vi "AlliGator FLI Dataset Actions.vi"(0 "AlliGator Q Elements":T4[](array[typedef]), 1 "VI in":refnum<vi>, 2 "Script in":bool, 5 "AlliGator IV DVR in":refnum<data-value>, 7 "AlliGator Q Event in":T5=enum."GUI:Idle", 9 "Data":variant, 11 "error in (no error)":errorcluster, 12 "AlliGator Ctrl Refnums":T6) -> (3 "Script out":bool, 4 "Alligator Queue Elements":T4[](array[typedef]), 6 "AlliGator IV DVR out":refnum<data-value>, 10 "[Notebook Message]":T1[](array[typedef]) {"Message Style"."Text Alignment" items=["Left", "Right", "Center"]}, 15 "error out":errorcluster)   [LabVIEW 2021, in "AlliGator Action Engine.lvlib"]
doc: "Processes AlliGator FLI Dataset-related actions."
uses:
  AlliGator Action Engine.lvlib
  AlliGator Internal Variables v2.ctl
  <vilib>/vision/Image Controls.llb/IMAQ Image.ctl
  AlliGator Gate Image Set.ctl
  AlliGator FLI Dataset Type.ctl
  AlliGator Data Series Type.ctl
  AlliGator Dataset Channel.ctl
  AlliGator Gate Arithmetic.ctl
  AlliGator Displayed Image.ctl
  Image/Named ROI Description.ctl
  AlliGator Decay Metadata v3.ctl
  AlliGator Decay Background Subtraction Info.ctl
  AlliGator Baseline Subtraction Method.ctl
  Graphs/XY Graph/XY Graph Plot Shift Parameters.ctl
  Graphs/XY Graph/XY Graph Plot Shift Method.ctl
  AlliGator Decay Extrapolation Parameters.ctl
  Phasor/Calibration Phasor (m, phi).ctl
  Phasor/Phasor Reference Series.ctl
  Phasor/Phasor Calibration Map v2.ctl
  Phasor/Phasor (g, s).ctl
  AlliGator Raw Phasor Plot Data v4.ctl
  Phasor/Phasor Standard Deviation Options.ctl
  AlliGator Phasor Multi-Harmonic Data.ctl
  Phasor/Phasor Harmonic Data.ctl
  AlliGator Decay Fit Options & Parameters v2.ctl
  Fits/IRF(X)PSED/Decay Fit Options v2.ctl
  Fits/Decay Convolution/Decay Model.ctl
  Fits/Residual Type.ctl
  Fits/IRF(X)PSED/Fit Weights Type.ctl
  Fits/Non-linear Fitting Method v2.ctl
  Fits/Fit Calculation Method.ctl
  Fits/Non-linear Fitting Algorithm.ctl
  AlliGator Decay Fit Parameter Constraints 2.ctl
  Fits/IRF(X)PSED/Decay Fit Parameters In List.ctl
  Fits/IRF(X)PSED/MLE Baseline Offset Type.ctl
  AlliGator Decay Preprocessing Parameters.ctl
  Fits/IRF(X)PSED/Decay Fit Parameters & Derived Quantities List.ctl
  AlliGator Parameter Maps Data.ctl
  AlliGator Q Event.ctl
  AlliGator Ctrl Refnums.ctl
  AlliGator Other Ctrl Refnums.ctl
  AlliGator State Indicator.ctl
  AlliGator Main Window Tabs.ctl
  AlliGator Phasor Plot Ctrl Refnums.ctl
  AlliGator Phasor Graph Ctrl Refnums.ctl
  Phasor/Phasor Calibration Type.ctl
  AlliGator Dataset Ctrl Refnums.ctl
  AlliGator Registered Events Ctrl Refnums.ctl
  AlliGator Image Histogram Control Refnums.ctl
  Histograms/Linear Histogram Options.ctl
  Histograms/Histogram Bin Option.ctl
  Histograms/Histogram Bin Position.ctl
  AlliGator Decay Fit Map Control Refnums.ctl
  AlliGator Q Element.ctl
  Notebook/Notebook Message Object.ctl
  Rich Text Box/Text Formatting.ctl
  Rich Text Box/Text Colors.ctl
  AlliGator State Indicators List.ctl
  Alligator Elements Order in Action Stack.ctl
  Graphs/Plot Point Style.ctl
  Graphs/LabVIEW Plot Interpolation.ctl
  AlliGator Channel Arithmetic Action Parameters.ctl
  AlliGator Multi-ROIs Dialog Type.ctl
  Image/Image Control ROI Description.ctl
  5f8aefbb-6789-42e2-90c6-aefb61e4d968.vi
  AlliGator Add Action Array to Stack.vi
  Variant/Variant to Data/Variant to Boolean.vi
  Graphs/XY Graph/XY Graph Add Single Plot with Name.vi
  Variant/Variant to Data/Variant to String.vi
  Image/Image.lvlib
  AlliGator ROIs.lvlib
  Variant/Variant.lvlib
  Variant/Variant to Data/Variant to Data.lvlib
  GUI/GUI.lvlib
  AlliGator Settings.lvlib
  AlliGator Dual-Channel Datasets.lvlib
  AlliGator Python Plugins.lvlib
  Sound/Sound.lvlib
  AlliGator Source Image.lvlib
  AlliGator Scripts.lvlib
  AlliGator IRF.lvlib
  AlliGator GUI.lvlib
  AlliGator Decay Fit.lvlib
  AlliGator Decay Statistics.lvlib
  AlliGator Internal Variables.lvlib
  AlliGator Decay Processing.lvlib
  Error/Error.lvlib
  AlliGator Decay Fit Parameter Map.lvlib
  AlliGator Phasor Graph.lvlib
  Graphs/Graphs.lvlib
  Graphs/XY Graph/XY Graph Add-Ons.lvlib
  Rich Text Box/Rich Text Box.lvlib
  Phasor/Phasor.lvlib
  AlliGator Decay Preprocessing.lvlib
  AlliGator Files.lvlib
  AlliGator Phasor Plot.lvlib
  Fits/Fits.lvlib
  Histograms/Histogram Window.lvlib
  Notebook/Notebook.lvlib
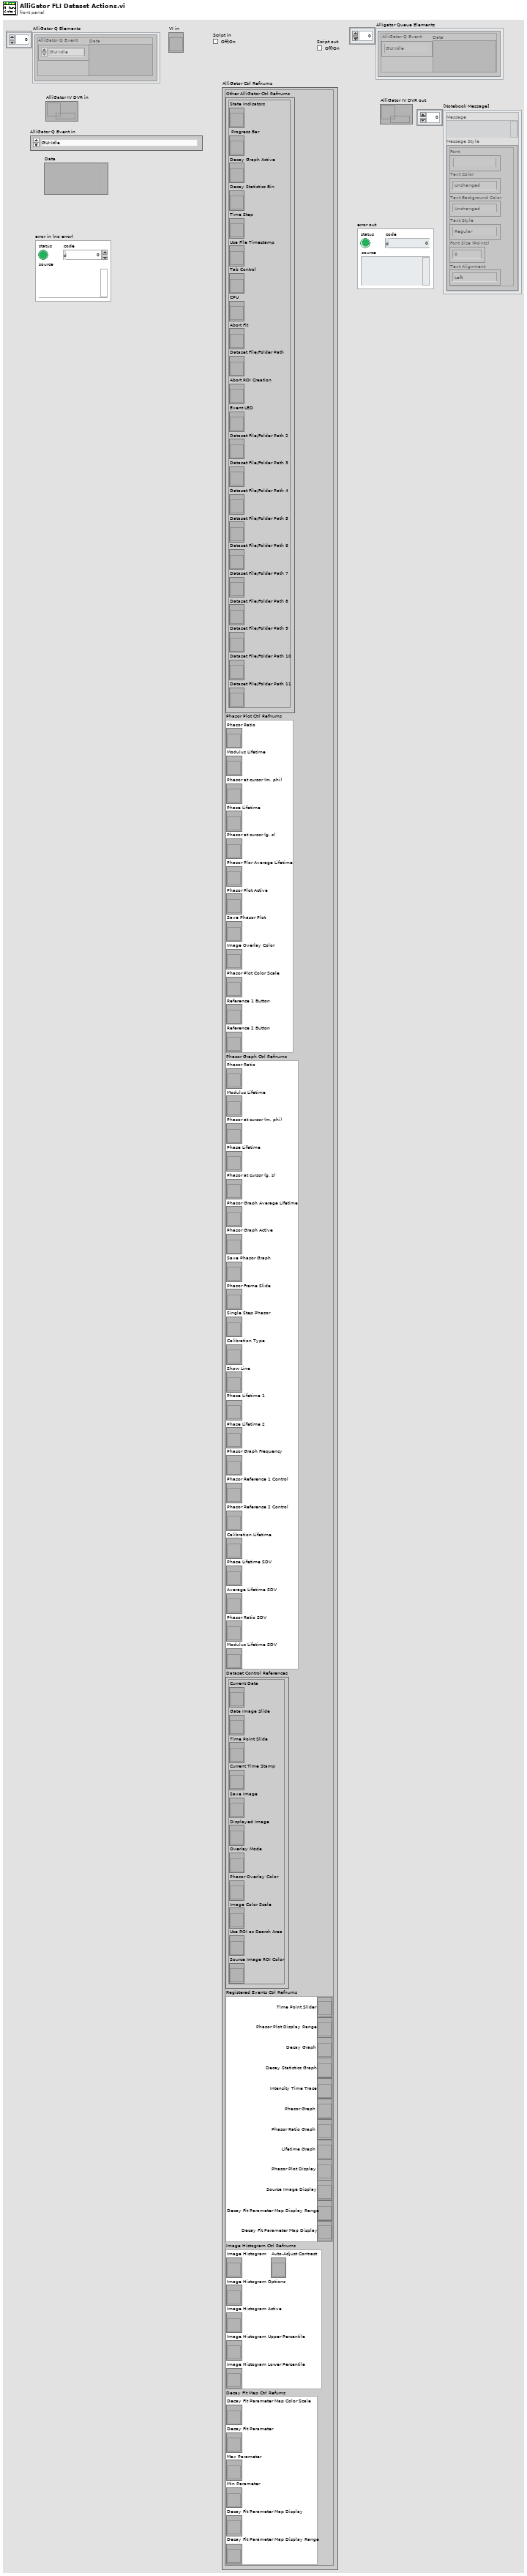
[diagram p1: front panel]
types:
  T1 = typedef "Notebook.lvlib/Notebook Message Object.ctl" = cluster{"Message":string, "Message Style":T2}
  T2 = typedef "Rich Text Box.lvlib/Text Formatting.ctl" = cluster{"Font":string, "Text Color":T3, "Text Background Color":T3, "Text Style":enum16{"Regular", "Bold", "Italic", "Underline", "Strikeout"}, "Font Size (Points)":dbl, "Text Alignment":i32}
  T3 = typedef "Rich Text Box.lvlib/Text Colors.ctl" = enum16{"Unchanged", "Black", "Blue", "Brown", "Gray", "Green", "Orange", "Pink", "Red", "White"}
  T4 = typedef "AlliGator Action Engine.lvlib/AlliGator Q Element.ctl" = cluster{"AlliGator Q Event":T5, "Data":variant}
  T5 = typedef "AlliGator Action Engine.lvlib/AlliGator Q Event.ctl" = enum16{"---- Files ----", "Files:Set Batch Export Files To Save", "Files:Set Dataset Loading & Pre-processing Options", "Files:Check #Frames in Dataset", "Files:Increment Frame Index", "Files:Open Mask Image", "Files:Open White Light Image", "Files:Open Single Dataset", "Files:New Folder of Folders Selected", "Files:Load File (all Types)_Scriptable", "Files:Move Flattened Series to Folders Series", "Files:Select Folder", "Files:Load FLI Dataset", "Files:Load Swiss SPAD 1 Dataset", "Files:Load Swiss SPAD 2 Dataset", "Files:Load .sdt FLI Dataset", "Files:Load .ptu FLI Dataset", "Files:Load .bin FLI Dataset", "Files:Load Single Gate Image Folder", "Files:Load I/m/phi Dataset (deprecated)", "Files:Load Single Image", "Files:Subtract Background File", "Files:Export FLI Dataset", "Files:Load HDF5 FLI Dataset", "Files:Set Destination File Path", "Files:Save Mask Image", "Files:Batch Conversion", "Files:New Folder Selected", "Files:Close FLI Dataset", "Files:Close FLI Dataset Series", "Files:Close White Light Image", "Files:Close Mask Image", "---- FLI Dataset ----", "FLI Dataset:Channel Arithmetic", "FLI Dataset:Export Average Lifetime Map as ASCII", "FLI Dataset:Export User-Defined Quantity Map as ASCII", "FLI Dataset:Python Function FLI Dataset Event", "FLI Dataset:ROI Analysis", "FLI Dataset:Tilted Logistic Square Gated IRF Characteristics Map", "FLI Dataset:Logistic Square Gated IRF Characteristics Map", "FLI Dataset:Square Gated IRF Characteristics Map", "FLI Dataset:Multi-ROI Single-Pixel Phasor Analysis", "FLI Dataset:Multi-ROI Single-Pixel NLSF Analysis", "FLI Dataset:All ROIs IRF Extraction", "FLI Dataset:All ROIs Decay Fit Non-Interactive (Fast + Individual IRF)", "FLI Dataset:All ROIs Phasor Analysis", "FLI Dataset:All ROIs Decay Fit", "FLI Dataset:Fluorescence Decay Statistics", "FLI Dataset:Update Decay Statistics Graph", "FLI Dataset:Get Decay from ROI", "FLI Dataset:All ROIs Average Lifetimes", "---- FLI Dataset Series ----", "FLI Dataset Series:Sum All Datasets in Series", "FLI Dataset Series:Add Dataset to Accumulated Dataset", "FLI Dataset Series:Display Accumulated Dataset", "FLI Dataset Series:Clear Dataset Series Sum", "FLI Dataset Series:Time-Series Analysis (NLSF)", "FLI Dataset Series:Time-Series Analysis (Phasor)", "---- Image ----", "Image:Update Image Profile Plots", "Image:Image Histogram Cursor Move", "Image:Image Histogram", "Image:Image Contrast", "Image:Set Image Histogram Cursor Move Flag", "Image:Clear Image Overlay", "Image:Use ROI as Search Area", "Image:Set ROI Diameter", "Image:Save Image Data as TIFF", "Image:Save Displayed Image with Overlay", "Image:Save Image Overlay Only", "Image:Save Image as Hot Pixel Mask", "Image:Change Source Image Color Palette", "Image:Copy Image to Clipboard", "Image:Source Image ROI Selection", "Image:Delete All ROIs", "Image:Delete All Unselected ROIs", "Image:Delete ROI", "Image:Merge All ROIs", "Image:Store ROI", "Image:Source Image ROI Storage", "Image:Export ROI Description to Notebook", "Image:Save ROI", "Image:Load ROI", "Image:Paste ROI Definition", "Image:Clear ROI", "Image:Identify ROIs in Mask Image", "Image:Create Complementary ROI", "Image:Create Contour ROI", "Image:Create ROI(s) from Pixels with Peak above Min_Scriptable", "Image:Create ROI(s) from Pixels with Intensity above Min_Scriptable", "Image:Compute ROI Statistics", "Image:Delete ROI(s) based on ROI Characteristics", "Image:Create ROI Grid", "Image:ROI to Individual Pixel ROIs", "Image:Python Function Source Image Event", "Image:Show Phasor Calibration Map ROI Centers", "Image:Convert ROI to Mask Image", "Image:Mouse Move", "Image:Mouse Up", "Image:Set Source Image Mouse Move Flag", "Image:Add Scale Bar Overlay", "Image:Delete Existing ROIs Option", "---- Decay ----", "Decay:Clear IRF/Reference Plot", "Decay:Clear Local IRFs", "Decay:Add Decay to Graph", "Decay:Smoothen Plot", "Decay:Smoothen Plot Tail", "Decay:Average Selected Plots", "Decay:Extract IRF", "Decay:Optimal IRF Extraction", "Decay:Threshold IRF", "Decay:Fit to Model IRF", "Decay:Fit IRF to Square Gate", "Decay:Fit IRF to Logistic Square Gate", "Decay:Fit IRF to Tilted Logistic Square Gate", "Decay:Create Bounding Cursors Set", "Decay:Export Bounding Cursors Definition to Notebook", "Decay:Denoise Plot", "Decay:Compute Cumulative Function", "Decay:Use as Reference Decay", "Decay:Show Reference Decay/IRF", "Decay:Extrapolate Decay", "Decay:Create Head & Tail Bounding Cursors", "Decay:Store Cursor-defined Head & Tail Fractions", "Decay:Rebin Plot", "Decay:1-Normalize Decay", "Decay:[0-1]-Normalize Plot", "Decay:Straighten Decay", "Decay:Shift Decay", "Decay:Fold Decay", "Decay:Fit Decay", "Decay:Global Fit of Selected Decays", "Decay:Post Global Fit Script", "Decay:Add Global Fit Parameters to Graph", "Decay:Add Decay Parameter(s) to Plot (Graph)", "Decay:Export Decay to Phasor Graph", "Decay:Plot Decay Shifts", "Decay:Compute Average Lifetime", "Decay:Plot Convolution", "Decay:Graph Tip Strip Update", "---- Decay Statistics ----", "Decay Statistics:Tip Strip Update", "---- Intensity Time Trace ----", "Intensity Time Trace:Use File Timestamp", "Intensity Time Trace:Load Intensity Corrections File", "Intensity Time Trace:Clear Intensity Corrections File", "Intensity Time Trace:Tip Strip Update", "---- Phasor Plot ----", "Phasor Plot:Build Phasor Plot", "Phasor Plot:Change Phasor Plot Color Palette", "Phasor Plot:Adjust Phasor Plot Display Range", "Phasor Plot:Highlight Image ROI in Phasor Plot", "Phasor Plot:Save Phasor Plot Image with Overlay", "Phasor Plot:Export Complex Phasor Map", "Phasor Plot:Export Phasor Ratio Map", "Phasor Plot:Export Average Lifetime Map", "Phasor Plot:Compute Phase Lifetime Histogram", "Phasor Plot:Compute Phasor Ratio Histogram", "Phasor Plot:Compute Phase Lifetime vs Intensity Scatter Plot", "Phasor Plot:Weber 2-Component Decomposition", "Phasor Plot:Update Phasor Color Map Vertices", "Phasor Plot:Clear Phasor Overlay", "Phasor Plot:Use Segment Extremities as References", "Phasor Plot:Use UC/Segment Intersections as References", "Phasor Plot:Use UC/Principal Axis Intersections as References", "Phasor Plot:Use UC/Linear Fit Intersections as References", "Phasor Plot:Update Phasor Plot Reference", "Phasor Plot:Show Local Phasor Info in Phasor Plot", "Phasor Plot:Update Phasor Plot State", "Phasor Plot:Phasor Plot ROI Storage", "Phasor Plot:Phasor Plot ROI Selection", "Phasor Plot:Python Function Phasor Plot Event", "Phasor Plot:Overlay Phasor ROI, Ratio or Map in Source Image", "Phasor Plot:Compute Decay of Selected Phasors", "Phasor Plot:Phasor at Image Pixel", "Phasor Plot:Mouse Move", "Phasor Plot:Mouse Up", "Phasor Plot:Display Range Mouse Move", "Phasor Plot:Set Mouse Move Flag", "---- Phasor Graph ----", "Phasor Graph:Calibrated Phasor Map Series", "Phasor Graph:Whole Image Phasor Scatter Plot (Todo)", "Phasor Graph:Get Phasor Value", "Phasor Graph:Create New Phasor Plot Dialog", "Phasor Graph:Update Last Phasor Value", "Phasor Graph:Update Phasor (m, phi)", "Phasor Graph:Remove Single Phasor from Plot", "Phasor Graph:Add Single Phasor to Plot", "Phasor Graph:Remove Phasor Plot", "Phasor Graph:Remove Selected Phasor Plots", "Phasor Graph:Clear Phasor Data", "Phasor Graph:Clear Phasor Graph", "Phasor Graph:Cursor Move", "Phasor Graph:Draw Cursor Connecting Line", "Phasor Graph:Clear Cursor Connecting Line", "Phasor Graph:Find UC Intersection", "Phasor Graph:Use UC/Cursor-Defined Line Intersections", "Phasor Graph:Use Selected Plots Fitted Line/UC Intersections", "Phasor Graph:Use Selected Plots Principal Axis/UC Intersections", "Phasor Graph:Show Single Phasor", "Phasor Graph:Save Single Phasor Plot", "Phasor Graph:Save All Phasor Plots", "Phasor Graph:Load Phasor Plot(s)", "Phasor Graph:Phasor Multiplication", "Phasor Graph:Compute Average Phasor", "Phasor Graph:Compute Multiple Average Phasors (Selected Plots)", "Phasor Graph:Export Single Phasor Plot Phase Lifetimes", "Phasor Graph:Phase Lifetime Trajectory", "Phasor Graph:Phase Lifetime vs Intensity Scatter Plot (deprecated)", "Phasor Graph:Parameter 2 vs Parameter 1 Scatter Plot", "Phasor Graph:Use Cursor n Location", "Phasor Graph:Set Reference n to Current Phase Lifetime Value", "Phasor Graph:Set Reference n to Lifetime Value", "Phasor Graph:Set Cursor n Location", "Phasor Graph:Save Phasor Graph Image", "Phasor Graph:Update SEPL Plot", "Phasor Graph:Export Single Phasor Plot Data", "Phasor Graph:Export Selected Phasor Plots Data", "Phasor Graph:Python Function Phasor Graph Event", "Phasor Graph:Tip Strip Update", "---- Calibration ----", "Calibration:Set Calibration Type", "Calibration:Load/Save Phasor Calibration", "Calibration:Load/Save Phasor Calibration Series", "Calibration:Load/Save Phasor Calibration Map", "Calibration:Use as Calibration", "Calibration:Compute Optimal Calibration from Phasor References", "Calibration:Clear Phasor Calibration", "Calibration:Single Phasor Calibration Information", "Calibration:Use as Calibration Series", "Calibration:Use as Calibration Map", "Calibration:Clear Calibration Series", "Calibration:Phasor Calibration Series Information", "Calibration:Clear Calibration Map", "Calibration:Phasor Calibration Map Information", "Calibration:Apply Phasor Calibration", "Calibration:Update Single Plot Calibration", "Calibration:Update Multiple Plots Calibration", "Calibration:Clear Single Plot Calibration", "Calibration:Clear All Plots Calibrations", "Calibration:Clear Plot(s) Calibration(s)?", "Calibration:Phasor Calibration Maps (# Gates Series)", "---- Phasor Ratio ----", "Phasor Ratio:Clear Reference n", "Phasor Ratio:Toggle Selected Plot(s)  Lock to Reference 1", "Phasor Ratio:Use as Reference n", "Phasor Ratio:Send Reference n to Notebook", "Phasor Ratio:Toggle Selected Plot(s)  Lock to Reference 2", "Phasor Ratio:Compute Phasor Ratio at Mouse Location", "Phasor Ratio:Compute Phasor Plot's Average Phasor Ratio", "Phasor Ratio:Compute Time-Series Phasor Ratios", "Phasor Ratio:Fit Line to Phasor Ratio Plot", "Phasor Ratio:Save References", "Phasor Ratio:Load References", "Phasor Ratio:Update Phasor Reference 1", "Phasor Ratio:Update Phasor Reference 2", "Phasor Ratio:Move Cursor n to Reference n", "Phasor Ratio:Use as Phasor Reference 1 Lifetime", "Phasor Ratio:Use as Phasor Reference 2 Lifetime", "Phasor Ratio:Export Phasor Ratio Map as ASCII", "Phasor Ratio:Tip Strip Update", "---- Lifetime & Other Parameters Graph ----", "Lifetime:Tip Strip Update", "---- Decay Fit Parameter Map ----", "Decay Fit Parameter Map:Export ROI NLSF Data as ASCII", "Decay Fit Parameter Map:Set Decay Fit  Parameter Map Selection", "Decay Fit Parameter Map:Build Decay Fit Parameter Map", "Decay Fit Parameter Map:Change Decay Fit Parameter Map Color Palette", "Decay Fit Parameter Map:Export Decay Fit Parameter Map Data as ASCII", "Decay Fit Parameter Map:Export All Decay Fit Parameter Maps Data as ASCII", "Decay Fit Parameter Map:Send Map Data to Lifetime Graph", "Decay Fit Parameter Map:Save Decay Fit Parameter Map Image", "Decay Fit Parameter Map:Save-Load IRFs & Fit Data", "Decay Fit Parameter Map:Update Local Decay Plots", "Decay Fit Parameter Map:Python Function Decay Fit Parameters Map Event", "Decay Fit Parameter Map:Overlay Decay Fit Parameter Map in Source Image", "Decay Fit Parameter Map:Plot Map Data vs Intensity", "Decay Fit Parameter Map:Mouse Up", "Decay Fit Parameter Map:Display Range Mouse Move", "---- Generic Graph ----", "Generic Graph:Generic XY Graph Event", "Generic Graph:Python Function XY Graph Event", "Generic Graph:New Plot", "Generic Graph:Save Plot", "Generic Graph:XY Plot Histogram", "Generic Graph:Set XY Graph Plot Name", "Generic Graph:Set Last Cursor Style", "Generic Graph:Tip Strip Update", "---- GUI ----", "GUI:Start Script", "GUI:Type of Displayed Image Changed", "GUI:Gate Image Slide Changed", "GUI:Show Busy Icon", "GUI:Show Busy Icon & Abort Button", "GUI:Hide Busy Icon", "GUI:Hide Busy Icon & Abort Button", "GUI:Abort", "GUI:End Script", "GUI:Start Timing", "GUI:End Timing", "GUI:Set State Indicator", "GUI:Send Parameters JSON Strings to Clipboard", "GUI:Set Gate Step", "GUI:Idle", "GUI:Initialization", "GUI:Quit", "GUI:Increment Dataset Index", "GUI:Set Dataset Index to -1", "GUI:Time Series Slider Moved", "GUI:Time Series Slider Changed", "GUI:Toggle Playback or Loop", "GUI:Playback Script", "GUI:Set Phasor Frequency", "GUI:Open Window", "GUI:Start Test Script", "GUI:End Test Script", "DEBUG"}
  T6 = typedef "AlliGator GUI.lvlib/AlliGator Ctrl Refnums.ctl" = cluster{"Other AlliGator Ctrl Refnums":T7, "Phasor Plot Ctrl Refnums":T8, "Phasor Graph Ctrl Refnums":T9, "Dataset Control References":T10, "Registered Events Ctrl Refnums":T11, "Image Histogram Ctrl Refnums":T12, "Decay Fit Map Ctrl Refums":T13}
  T7 = typedef "AlliGator GUI.lvlib/AlliGator Other Ctrl Refnums.ctl" = cluster{"State Indicators":refnum<vi>, " Progress Bar":refnum<vi>, "Decay Graph Active":refnum<vi>, "Decay Statistics Bin":refnum<vi>, "Time Step":refnum<vi>, "Use File Timestamp":refnum<vi>, "Tab Control":refnum<vi>, "CPU":refnum<vi>, "Abort Fit":refnum<vi>, "Dataset File/Folder Path":refnum<vi>, "Abort ROI Creation":refnum<vi>, "Event LED":refnum<vi>, "Dataset File/Folder Path 2":refnum<vi>, "Dataset File/Folder Path 3":refnum<vi>, "Dataset File/Folder Path 4":refnum<vi>, "Dataset File/Folder Path 5":refnum<vi>, "Dataset File/Folder Path 6":refnum<vi>, "Dataset File/Folder Path 7":refnum<vi>, "Dataset File/Folder Path 8":refnum<vi>, "Dataset File/Folder Path 9":refnum<vi>, "Dataset File/Folder Path 10":refnum<vi>, "Dataset File/Folder Path 11":refnum<vi>}
  T8 = typedef "AlliGator GUI.lvlib/AlliGator Phasor Plot Ctrl Refnums.ctl" = cluster{"Phasor Ratio":refnum<vi>, "Modulus Lifetime":refnum<vi>, "Phasor at cursor (m, phi)":refnum<vi>, "Phase Lifetime":refnum<vi>, "Phasor at cursor (g, s)":refnum<vi>, "Phasor Plor Average Lifetime":refnum<vi>, "Phasor Plot Active":refnum<vi>, "Save Phasor Plot":refnum<vi>, "Image Overlay Color":refnum<vi>, "Phasor Plot Color Scale":refnum<vi>, "Reference 1 Button":refnum<vi>, "Reference 2 Button":refnum<vi>}
  T9 = typedef "AlliGator GUI.lvlib/AlliGator Phasor Graph Ctrl Refnums.ctl" = cluster{"Phasor Ratio":refnum<vi>, "Modulus Lifetime":refnum<vi>, "Phasor at cursor (m, phi)":refnum<vi>, "Phase Lifetime":refnum<vi>, "Phasor at cursor (g, s)":refnum<vi>, "Phasor Graph Average Lifetime":refnum<vi>, "Phasor Graph Active":refnum<vi>, "Save Phasor Graph":refnum<vi>, "Phasor Frame Slide":refnum<vi>, "Single Step Phasor":refnum<vi>, "Calibration Type":refnum<vi>, "Show Line":refnum<vi>, "Phase Lifetime 1":refnum<vi>, "Phase Lifetime 2":refnum<vi>, "Phasor Graph Frequency":refnum<vi>, "Phasor Reference 1 Control":refnum<vi>, "Phasor Reference 2 Control":refnum<vi>, "Calibration Lifetime":refnum<vi>, "Phase Lifetime SDV":refnum<vi>, "Average Lifetime SDV":refnum<vi>, "Phasor Ratio SDV":refnum<vi>, "Modulus Lifetime SDV":refnum<vi>}
  T10 = typedef "AlliGator GUI.lvlib/AlliGator Dataset Ctrl Refnums.ctl" = cluster{"Current Data":refnum<vi>, "Gate Image Slide":refnum<vi>, "Time Point Slide":refnum<vi>, "Current Time Stamp":refnum<vi>, "Save Image":refnum<vi>, "Displayed Image":refnum<vi>, "Overlay Mode":refnum<vi>, "Phasor Overlay Color":refnum<vi>, "Image Color Scale":refnum<vi>, "Use ROI as Search Area":refnum<vi>, "Source Image ROI Color":refnum<vi>}
  T11 = typedef "AlliGator GUI.lvlib/AlliGator Registered Events Ctrl Refnums.ctl" = cluster{"Time Point Slider":refnum<vi>, "Phasor Plot Display Range":refnum<vi>, "Decay Graph":refnum<vi>, "Decay Statistics Graph":refnum<vi>, "Intensity Time Trace":refnum<vi>, "Phasor Graph":refnum<vi>, "Phasor Ratio Graph":refnum<vi>, "Lifetime Graph":refnum<vi>, "Phasor Plot Display":refnum<vi>, "Source Image Display":refnum<vi>, "Decay Fit Parameter Map Display Range":refnum<vi>, "Decay Fit Parameter Map Display":refnum<vi>}
  T12 = typedef "AlliGator GUI.lvlib/AlliGator Image Histogram Control Refnums.ctl" = cluster{"Image Histogram":refnum<vi>, "Image Histogram Options":refnum<vi>, "Image Histogram Active":refnum<vi>, "Image Histogram Upper Percentile":refnum<vi>, "Image Histogram Lower Percentile":refnum<vi>, "Auto-Adjust Contrast":refnum<vi>}
  T13 = typedef "AlliGator Decay Fit Parameter Map.lvlib/AlliGator Decay Fit Map Control Refnums.ctl" = cluster{"Decay Fit Parameter Map Color Scale":refnum<vi>, "Decay Fit Parameter":refnum<vi>, "Max Parameter":refnum<vi>, "Min Parameter":refnum<vi>, "Decay Fit Parameter Map Display":refnum<vi>, "Decay Fit Parameter Map Display Range":refnum<vi>}
  T14 = typedef "AlliGator Action Engine.lvlib/Alligator Elements Order in Action Stack.ctl" = enum16{"Enqueue 2 AFTER 1", "Enqueue 2 BEFORE 1"}
  T15 = typedef "AlliGator Action Engine.lvlib/AlliGator State Indicators List.ctl" = enum16{"Phasor Calibration Defined", "Phasor Calibration Series Defined", "Phasor Calibration Map Defined", "Phasor Reference 1 Defined", "Phasor Reference 2 Defined", "Lifetime Reference 1 Defined", "Lifetime Reference 2 Defined", "Phasor Calibration Used", "Phasor Calibration Series Used", "Phasor Calibration Map Used", "Dataset Update Needed", "Phasor Plot Update Needed", "Reference/IRF Defined", "Individual IRFs Defined"}
  T16 = typedef "Graphs.lvlib/Plot Point Style.ctl" = enum16{"not defined", "None", "Empty Circle", "Filled Circle", "Thick Circle", "Dotted Circle", "Empty Square", "Filled Square", "Thick Square", "Dotted Square", "Small Filled Square", "Dot", "Cross", "Tiny Cross", "Large X", "Small x", "Diamond", "Small Empty Square"}
  T17 = typedef "AlliGator Dual-Channel Datasets.lvlib/AlliGator Channel Arithmetic Action Parameters.ctl" = cluster{"Channel Name":u16, "Channel Arithmetic":T18}
  T18 = typedef "AlliGator Settings.lvlib/AlliGator Gate Arithmetic.ctl" = enum16{"None", "INT-G2", "G2/INT*<INT>", "(1 - G2/INT)*<INT>"}
  T19 = typedef "ROI Descriptor" = cluster{"Global Rectangle":i32[], "Contours":cluster{"ID":enum32{"External", "Internal"}, "Type":u32, "Coordinates":i32[]}[]}
  T20 = typedef "AlliGator Scripts.lvlib/AlliGator Multi-ROIs Dialog Type.ctl" = enum16{"Multi-ROIs Single-Pixel Phasor Analysis", "Multi-ROIs Single-Pixel NLSF Analysis", "Export ROI Fit Parameters as ASCII"}
  T21 = typedef "Image.lvlib/Image Control ROI Description.ctl" = cluster{"Image Control Label":string, "ROI Descriptor":T19}
  T22 = typedef "AlliGator GUI.lvlib/AlliGator State Indicator.ctl" = cluster{"Phasor Calibration Defined":bool, "Phasor Calibration Series Defined":bool, "Phasor Calibration Map Defined":bool, "Phasor Ratio Reference 1 Defined":bool, "Phasor Ratio Reference 2 Defined":bool, "Phasor Ratio Lifetime Reference 1 Defined ":bool, "Phasor Ratio Lifetime Reference 2 Defined":bool, "Phasor Calibration Used":bool, "Phasor Calibration Series Used":bool, "Phasor Calibration Map Used":bool, "Dataset Update Needed":bool, "Phasor Plot Update Needed":bool, "Reference/IRF Defined":bool, "Individual IRFs Defined":bool}
  T23 = typedef "Graphs.lvlib/LabVIEW Plot Interpolation.ctl" = u8
  T24 = typedef "IMAQ Image.ctl" = refnum<image>
  T25 = typedef "AlliGator Scripts.lvlib/AlliGator Data Load & Process Options.ctl" = cluster{"Data Information":T26, "Source Image Settings":T30, "Decay Preprocessing Options & Parameters":T37, "Clear Phasor Graph":bool}
  T26 = typedef "AlliGator Scripts.lvlib/AlliGator Data Information.ctl" = cluster{"Gates to Skip":T27, "# Gates":u32, "Gate Step":u32, "Gate Duration":dbl[unit], "Gate Separation":dbl[unit], "Pile-up Correction":bool, "Pixel Well Capacity":u32, "Define Gates to":T28, "Gates to Keep":T29, "Laser Period":dbl[unit], "SYNC Period":dbl[unit], "Channel Name":u16, "Channel Arithmetic":T18, "Background File Subtraction":bool, "Background Scaling Factor":dbl, "Background File":path, "Background Pile-up Correction":bool, "Background Pixel Well Capacity":u32, "Dataset Scaling Factor":dbl}
  T27 = typedef "AlliGator Decay Analysis.lvlib/AlliGator Gates to Skip.ctl" = cluster{"Start":u32, "End":u32}
  T28 = typedef "AlliGator Settings.lvlib/AlliGator Define Gates to.ctl" = enum32{"Skip", "Keep"}
  T29 = typedef "AlliGator Settings.lvlib/AlliGator Gates to Keep.ctl" = cluster{"First":u32, "Last":u32}
  T30 = typedef "AlliGator Scripts.lvlib/AlliGator Source Image Settings.ctl" = cluster{"Low Count Pixels Rejection Options":T31, "High Count Pixels Rejection Options":T32, "Peak Threshold":dbl, "Intensity Threshold":dbl, "Image Smoothing Options":T33, "Image Binning Options":T36}
  T31 = typedef "AlliGator Settings.lvlib/AlliGator Low Count Pixels Rejection Options.ctl" = cluster{"Background Low Threshold Factor":dbl, "Fixed Low Background Threshold":dbl, "Reject Low Count Pixels":bool, "Low Percentile":dbl}
  T32 = typedef "AlliGator Settings.lvlib/AlliGator High Count Pixels Rejection Options.ctl" = cluster{"Background High Threshold Factor":dbl, "Fixed High Background Threshold":dbl, "Reject High Count Pixels":bool, "High Percentile":dbl}
  T33 = typedef "AlliGator Settings.lvlib/AlliGator Image Smoothing Options.ctl" = cluster{"Use Image Smoothing":bool, "Kernel Type":T34, "Bin":i32, "Algorithm":T35}
  T34 = typedef "Arrays.lvlib/Kernel Type.ctl" = enum16{"Uniform", "Bilinear", "Gaussian"}
  T35 = typedef "Arrays.lvlib/Smoothing Algorithm.ctl" = enum16{"Rapid", "Thorough"}
  T36 = typedef "AlliGator Source Image.lvlib/AlliGator Image Binning Options.ctl" = cluster{"Use Image Binning":bool, "X Bin":i32, "Y Bin":i32}
  T37 = typedef "AlliGator Decay Analysis.lvlib/AlliGator Decay Preprocessing.lvlib/AlliGator Decay Preprocessing Options.ctl" = cluster{"Background Subtraction Parameters":T38, "Decay Preprocessing Parameters":T40, "Preprocessing Steps Order":string[]}
  T38 = typedef "AlliGator Decay Analysis.lvlib/AlliGator Decay Preprocessing.lvlib/AlliGator Background Subtraction Parameters.ctl" = cluster{"Background Definition Range":cluster{"Min Gate":dbl[unit], "Max Gate":dbl[unit]}, "Baseline Subtraction Method":T39, "Background Subtraction?":bool, "Background File":path, "Background Constant":dbl, "Background Scaling Factor":dbl, "Background Pile-up Correction":bool, "Background Pixel Well Capacity":u32}
  T39 = typedef "AlliGator Decay Analysis.lvlib/AlliGator Decay Preprocessing.lvlib/AlliGator Baseline Subtraction Method.ctl" = enum16{"Mean", "Min", "Square Gated Single-Exponential", "File", "Constant"}
  T40 = typedef "AlliGator Decay Analysis.lvlib/AlliGator Decay Preprocessing.lvlib/AlliGator Decay Preprocessing Parameters.ctl" = cluster{"Background Subtraction":bool, "Straighten Decay":bool, "Reverse Gates":bool, "1-Normalized Decay":bool, "Smoothen Decay":bool, "Smoothing Parameter":dbl, "Shift Decay":bool, "Decay Shift Parameters":T41, "Extrapolate Decay":bool, "Additional Points":u32, "Head Fraction":dbl, "Pixel-Normalize Decay":bool, "Use Periodicity":bool, "Use Cursors":bool, "Tail Fraction":dbl, "Use Decay Pre-Processing":bool, "Fold Decay":bool, "# Folds":u32, "[0-1]-Normalized Decay":bool}
  T41 = typedef "XY Graph Add-Ons.lvlib/XY Graph Plot Shift Parameters.ctl" = cluster{"Type":T42, "Shift":dbl[unit], "Threshold":dbl, "Rotate":bool}
  T42 = typedef "XY Graph Add-Ons.lvlib/XY Graph Plot Shift Method.ctl" = enum16{"Default", "CFD", "Threshold", "Cross-Correlation"}
  T43 = typedef "Fits.lvlib/Decay Fit Parameters & Derived Quantities List.ctl" = enum16{"Offset", "Baseline", "A_1", "tau_1", "A_2", "tau_2", "<tau>_a", "f1_a", "f2_a", "<tau>_i", "f1_i", "f2_i", "-", "R^2", "Chi^2"}
  T44 = typedef "AlliGator Phasor Graph.lvlib/AlliGator Phasor Plot Scatter Plot Parameters.ctl" = cluster{"Parameter 2":T45, "Parameter 1":T45}
  T45 = typedef "AlliGator Phasor Graph.lvlib/AlliGator Phasor Graph Parameter List.ctl" = enum16{"Time Stamp", "Index", "Phasor Parameters", "Phasor g", "Phasor s", "Phasor phi", "Phasor m", "Modulus Lifetime", "Phase Lifetime", "ROI Parameters", "ROI Center x", "ROI Center y", "ROI # pixels ", "Decay Parameters", "Intensity", "Background/Gate", "Intensity - Background", "Fitted Lifetime", "Fitted Intensity", "Phasor Ratio Parameters", "Amplitude Phasor Ratio", "Intensity Phasor Ratio", "Amplitude-Averaged Lifetime", "Intensity-Averaged Lifetime", "-", "Phasor Parameters SDV", "Phasor g SDV", "Phasor s SDV", "Phasor phi SDV", "Phasor m SDV", "Phase Lifetime SDV", "Modulus Lifetime SDV", "Phasor Ratio Parameters SDV", "Amplitude Phasor Ratio SDV", "Intensity Phasor Ratio SDV", "Amplitude-Averaged Lifetime SDV", "Intensity-Averaged Lifetime SDV"}
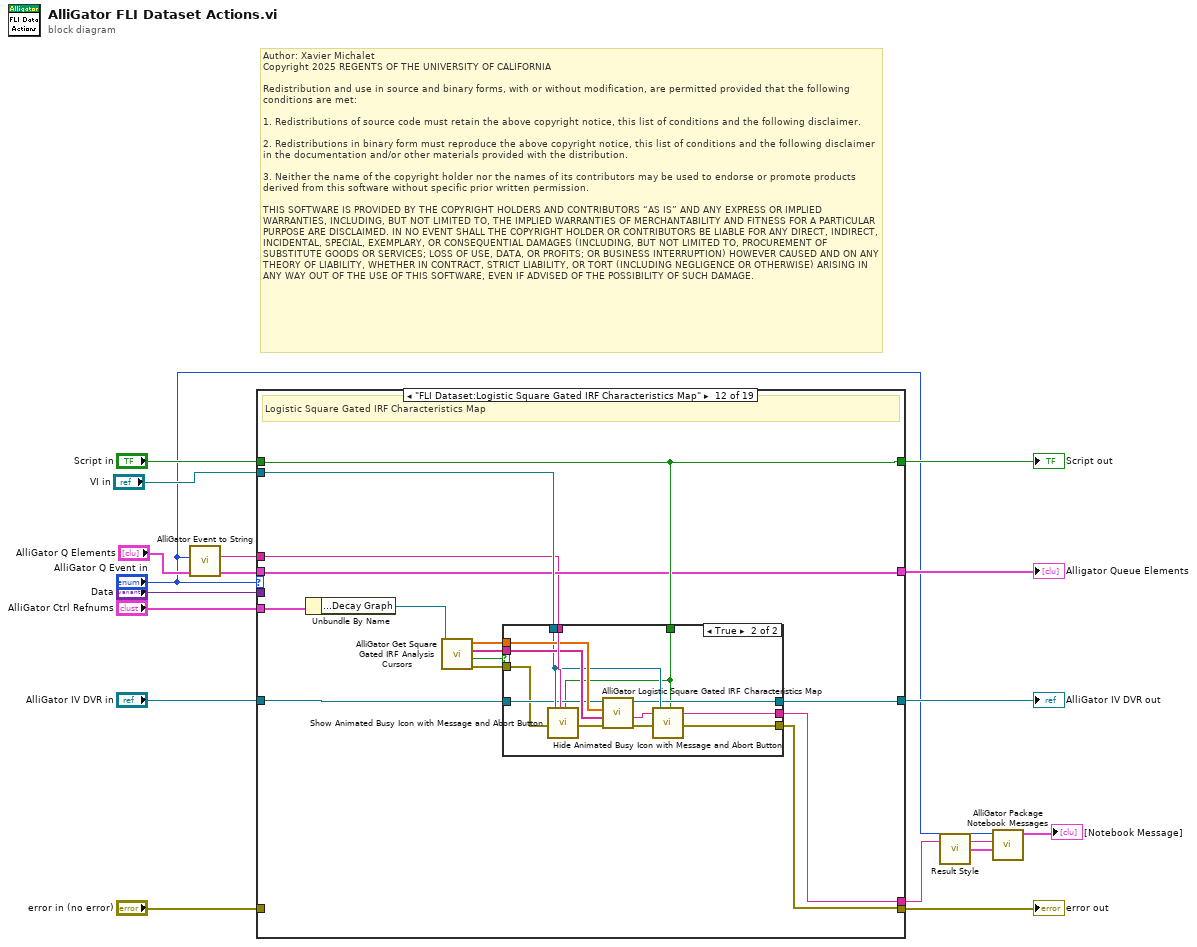
[diagram p0: block diagram]
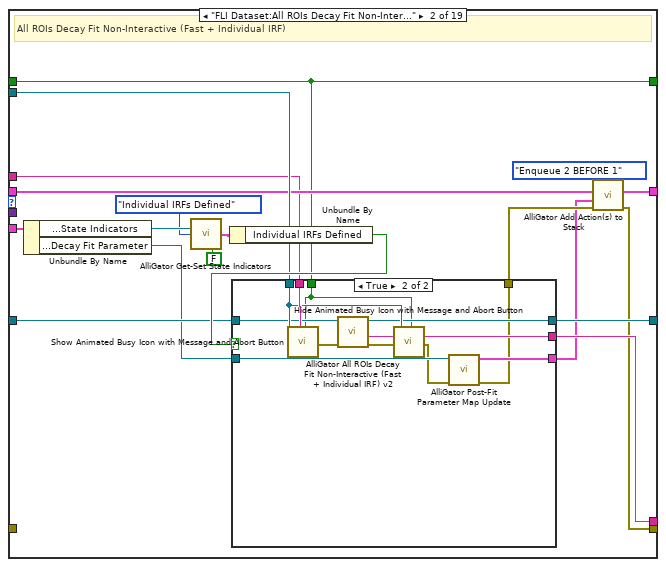
[diagram p3: hidden frame]
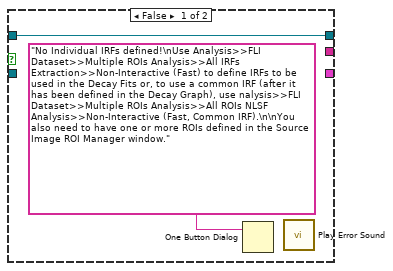
[diagram p4: hidden frame]
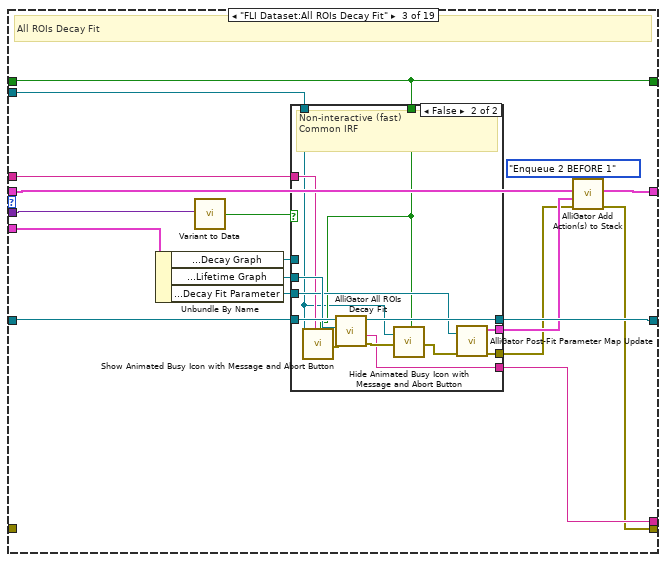
[diagram p5: hidden frame]
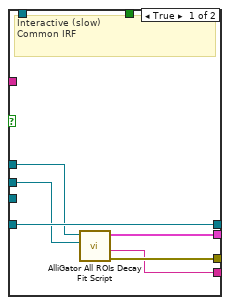
[diagram p6: hidden frame]
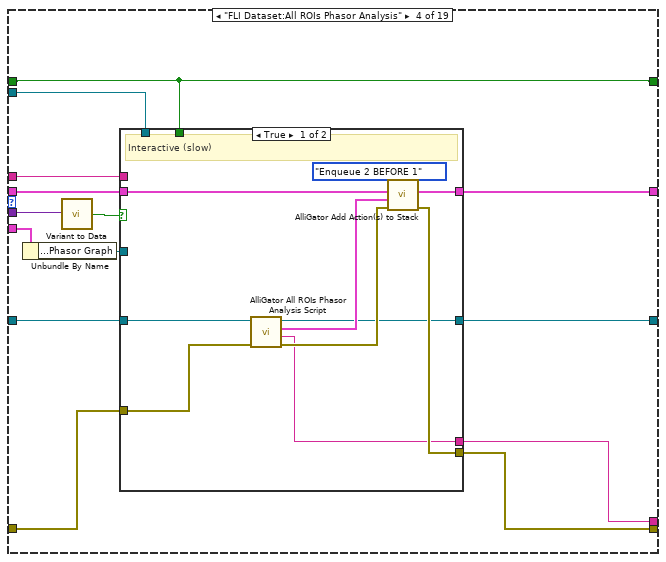
[diagram p7: hidden frame]
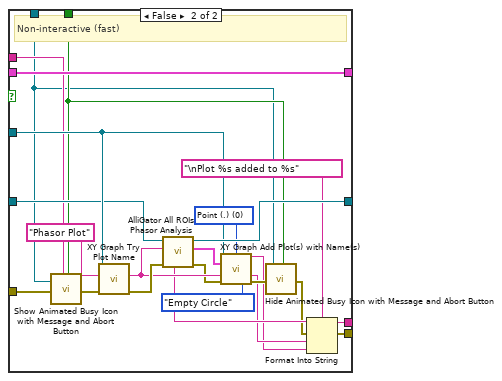
[diagram p8: hidden frame]
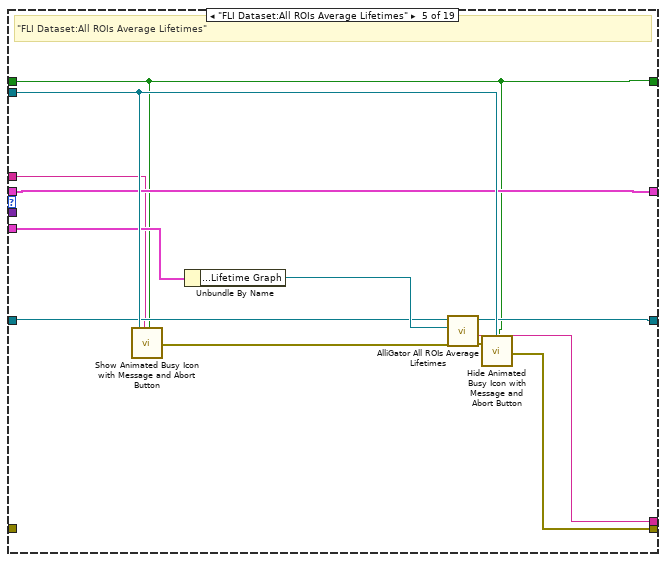
[diagram p9: hidden frame]
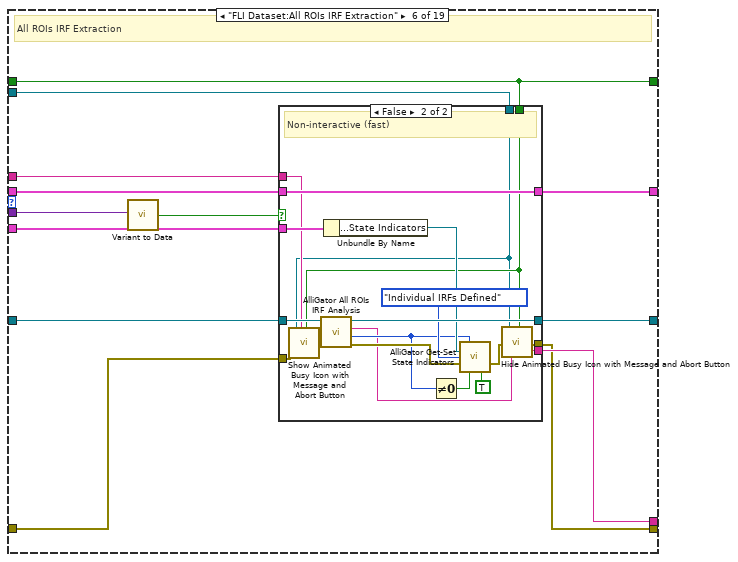
[diagram p10: hidden frame]
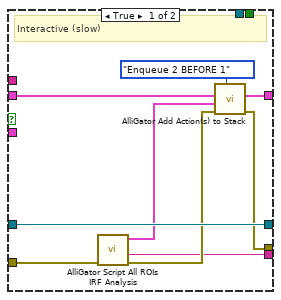
[diagram p11: hidden frame]
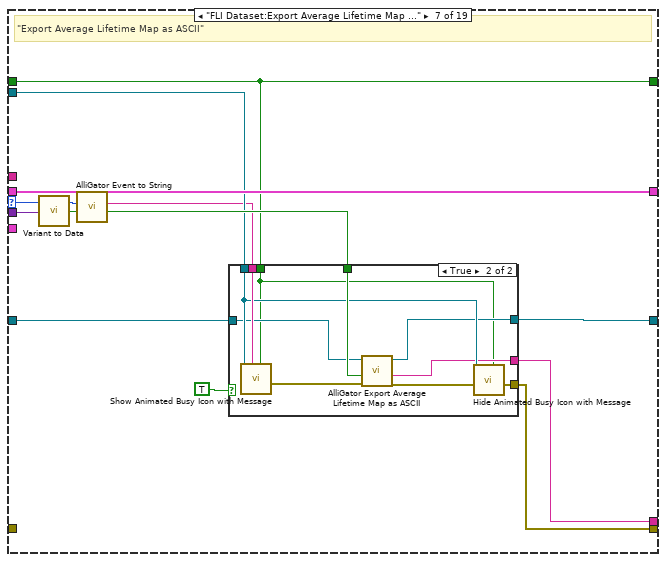
[diagram p12: hidden frame]
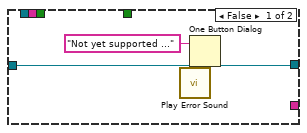
[diagram p13: hidden frame]
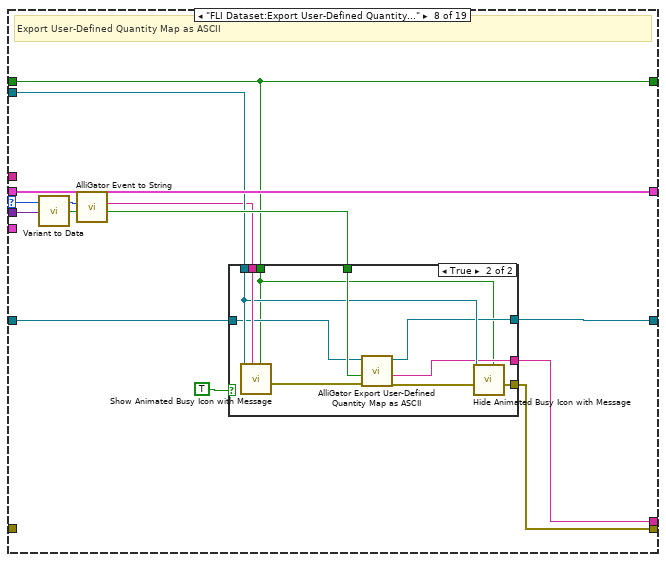
[diagram p14: hidden frame]
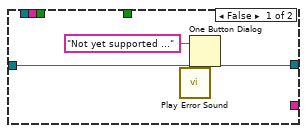
[diagram p15: hidden frame]
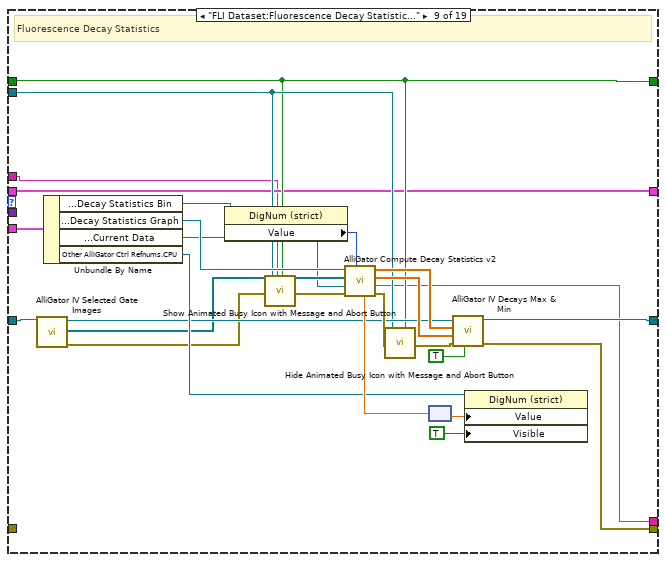
[diagram p16: hidden frame]
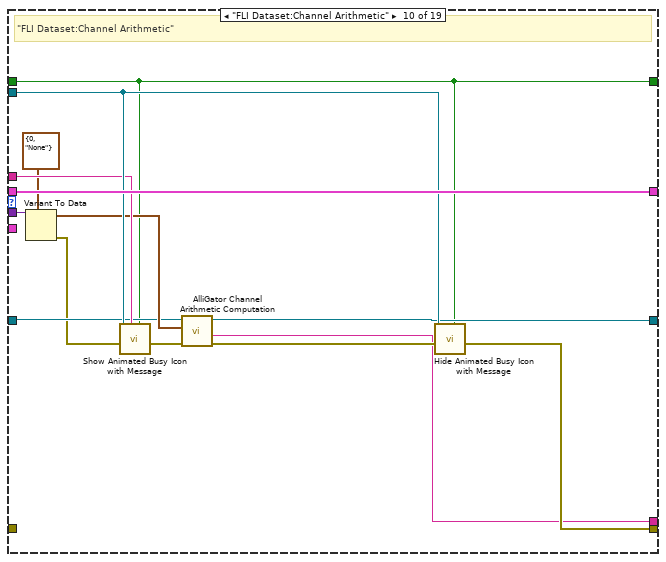
[diagram p17: hidden frame]
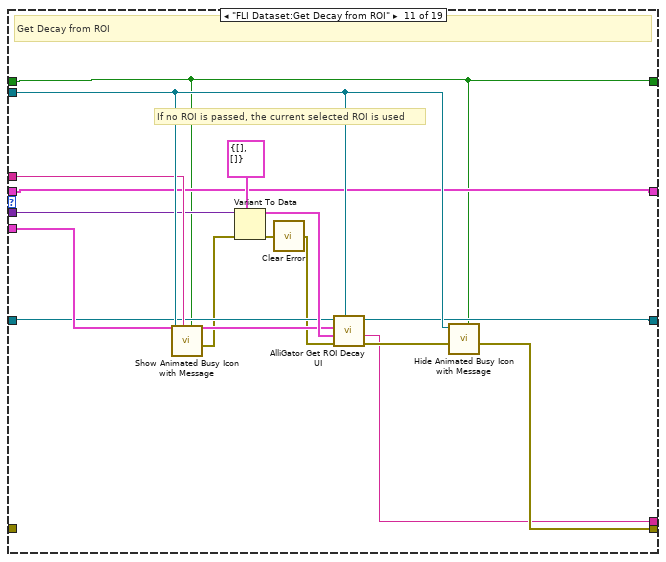
[diagram p18: hidden frame]
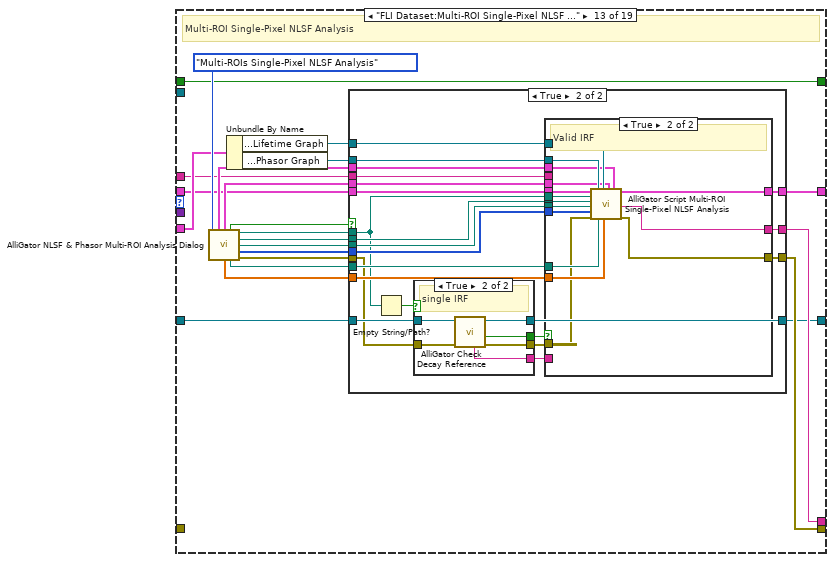
[diagram p20: hidden frame]
diagram:
  # "Author: Xavier Michalet\nCopyright 2025 REGENTS OF THE UNIVERSITY OF CALIFORNIA\n\nRedistribution and use in source and binary forms, with or without modification, are permitted provided that the following conditions are met:\n\n1. Redistributions of source code must retain the above copyright notice, this list of conditions and the following disclaimer.\n\n2. Redistributions in binary form must reproduce the above copyright notice, this list of conditions and the following disclaimer in the documentation and/or other materials provided with the distribution.\n\n3. Neither the name of the copyright holder nor the names of its contributors may be used to endorse or promote products derived from this software without specific prior written permission.\n\nTHIS SOFTWARE IS PROVIDED BY THE COPYRIGHT HOLDERS AND CONTRIBUTORS “AS IS” AND ANY EXPRESS OR IMPLIED WARRANTIES, INCLUDING, BUT NOT LIMITED TO, THE IMPLIED WARRANTIES OF MERCHANTABILITY AND FITNESS FOR A PARTICULAR PURPOSE ARE DISCLAIMED. IN NO EVENT SHALL THE COPYRIGHT HOLDER OR CONTRIBUTORS BE LIABLE FOR ANY DIRECT, INDIRECT, INCIDENTAL, SPECIAL, EXEMPLARY, OR CONSEQUENTIAL DAMAGES (INCLUDING, BUT NOT LIMITED TO, PROCUREMENT OF SUBSTITUTE GOODS OR SERVICES; LOSS OF USE, DATA, OR PROFITS; OR BUSINESS INTERRUPTION) HOWEVER CAUSED AND ON ANY THEORY OF LIABILITY, WHETHER IN CONTRACT, STRICT LIABILITY, OR TORT (INCLUDING NEGLIGENCE OR OTHERWISE) ARISING IN ANY WAY OUT OF THE USE OF THIS SOFTWARE, EVEN IF ADVISED OF THE POSSIBILITY OF SUCH DAMAGE."
  n1 = call "AlliGator Event to String.vi"("AlliGator Q Event"="AlliGator Q Event in") -> ("String"=w6:string)  [unwired: 8 in]
  n2 = case shown="\"FLI Dataset:Logistic Square Gated IRF Characteristics Map\"" "AlliGator Q Event in" {
    selector: "AlliGator Q Event in" -> [_ _ _ _ _ _ w193 w217 _ _ _ _ _ w399 _ _ _ _ _]
    tunnel: "Data" -> [_ _ w67 w97 _ w160 w201 w225 _ w275 w288 _ _ _ w437 _ _ _ _]
    tunnel: "AlliGator Q Elements" -> [w20 w33 w56 w102 w142 w161 w202 w226 w245 w278 w289 w301 w327 w403 w452 w477 w485 w494 w519]
    tunnel: [w20 w26 w62 w101 w142 w157 w202 w226 w245 w278 w289 w301 w329 w402 w451 w476 w485 w494 w519] -> w8
    tunnel: "VI in" -> [_ w34 w68 w96 w148 w162 w196 w220 w247 w277 w291 w303 _ _ w453 _ w484 w496 w523]
    tunnel: [w19 w21 w54 w91 w139 w151 w198 w222 w246 w265 w282 w302 w323 w404 w435 w470 w478 w495 w516] -> w9
    tunnel: "Script in" -> [w19 w21 w54 w91 w139 w151 w198 w222 w246 w265 w282 w302 w323 w404 w435 w470 w478 w495 w516]
    tunnel: w6 -> [_ w32 w55 w93 w141 w153 _ _ w244 w274 w290 w296 w326 _ w454 _ w483 w493 w517]
    tunnel: "error in (no error)" -> [w18 _ _ w92 _ w152 _ _ _ _ _ _ _ w397 _ _ _ _ _]
    tunnel: [w18 w23 w59 w95 w145 w154 w199 w223 w241 w273 w284 w297 w331 w400 w448 w469 w479 w490 w518] -> w5
    tunnel: "AlliGator Ctrl Refnums" -> [_ w31 w66 w94 w147 w159 _ _ w239 _ w287 w295 w328 w398 w442 w468 _ w492 w522]
    tunnel: "AlliGator IV DVR in" -> [w17 w30 w65 w100 w146 w158 w195 w219 w243 w270 w286 w300 w325 w418 w446 w455 w482 w491 w521]
    tunnel: [w17 w28 w63 w99 w143 w156 w194 w218 w242 w268 w285 w299 w324 w418 w445 w455 w481 w488 w520] -> w16
    tunnel: [_ w29 w64 w98 w144 w155 w191 w215 w240 w266 w283 w298 w330 w401 w443 _ w480 w489 _] -> w3
    frame "---- FLI Dataset ----", Default {
    }
    frame "FLI Dataset:All ROIs Decay Fit Non-Interactive (Fast + Individual IRF)" {
      # "All ROIs Decay Fit Non-Interactive (Fast + Individual IRF)"
      n3 = Unbundle By Name(w31) -> ("Other AlliGator Ctrl Refnums.State Indicators"=w39:refnum<vi>, "Decay Fit Map Ctrl Refums.Decay Fit Parameter"=w27:refnum<vi>)
      n4 = call "AlliGator Get-Set State Indicators.vi"("State Indicators Refnum"=w39, "AlliGator State Indicators List"=AlliGator_State_Indicators_List."Individual IRFs Defined", "Set (T)/Get"=FALSE) -> ("State Indicator Values"=w36:T22)  [unwired: 10 in, 2 out]
      n5 = Unbundle By Name(w36) -> ("Individual IRFs Defined"=w35:bool)
      n6 = case shown="True" w35 {
        tunnel: w32 -> [_ w53]
        tunnel: w21 -> [_ w48]
        tunnel: [_ w42] -> w25
        tunnel: w34 -> [_ w51]
        tunnel: w30 -> [w40 w50]
        tunnel: [w40 w49] -> w28
        tunnel: [_ w47] -> w29
        tunnel: w27 -> [_ w46]
        tunnel: [_ w44] -> w24
        frame False {
          n7 = One Button Dialog(message="No Individual IRFs defined!\nUse Analysis>>FLI Dataset>>Multiple ROIs Analysis>>All IRFs Extraction>>Non-Interactive (Fast) to define IRFs to be used in the Decay Fits or, to use a common IRF (after it has been defined in the Decay Graph), use nalysis>>FLI Dataset>>Multiple ROIs Analysis>>All ROIs NLSF Analysis>>Non-Interactive (Fast, Common IRF).\n\nYou also need to have one or more ROIs defined in the Source Image ROI Manager window.") -> ()  [unwired: 1 in, 1 out]
          n8 = call "Play Error Sound.vi"() -> ()  [unwired: 27 in, 1 out]
        }
        frame True {
          n9 = call "Show Animated Busy Icon with Message and Abort Button.vi"("Already active? (F)"=w48, "Message"=w53, "Target VI reference"=w51) -> ("Error Out"=w52:errorcluster)  [unwired: 16 in]
          n10 = call "AlliGator All ROIs Decay Fit Non-Interactive (Fast + Individual IRF) v2.vi"("error in (no error)"=w52, "AlliGator Internal Variables DVR"=w50) -> ("error out"=w45:errorcluster, "Message"=w47:string, "AlliGator Internal Variables DVR"=w49:refnum<data-value>)  [unwired: 7 in]
          n11 = call "Hide Animated Busy Icon with Message and Abort Button.vi"("Already active? (F)"=w48, "Target VI reference"=w51, "Error In"=w45) -> ("Error Out"=w43:errorcluster)  [unwired: 16 in]
          n12 = call "AlliGator Post-Fit Parameter Map Update.vi"("Error In"=w43, "Decay Fit Parameter"=w46) -> ("Error Out"=w42:errorcluster, "Array of Actions"=w44:T4[])  [unwired: 8 in]
        }
      }
      n13 = call-poly "AlliGator Add Action(s) to Stack.vi"("Elements Order in Action Stack (Default: 2 BEFORE 1)"=Alligator_Elements_Order_in_Action_Stack."Enqueue 2 BEFORE 1", "Error In"=w25, "Alligator Queue Element 2"=w24, "Alligator Queue Element 1"=w33) -> ("Error Out"=w23:errorcluster, "Alligator Queue Element 1 (+ 2)"=w26:T4[])  [unwired: 6 in]
    }
    frame "FLI Dataset:All ROIs Decay Fit" {
      # "All ROIs Decay Fit"
      n14 = Unbundle By Name(w66) -> ("Registered Events Ctrl Refnums.Decay Graph"=w70:refnum<vi>, "Registered Events Ctrl Refnums.Lifetime Graph"=w69:refnum<vi>, "Decay Fit Map Ctrl Refums.Decay Fit Parameter"=w58:refnum<vi>)
      n15 = call-poly "Variant to Data.vi"("Variant"=w67) -> ("Value"=w71:bool)  [unwired: 8 in]
      n16 = case shown="False" w71 {
        tunnel: w65 -> [w77 w90]
        tunnel: [w77 w89] -> w63
        tunnel: w68 -> [_ w79]
        tunnel: w54 -> [_ w81]
        tunnel: [w76 w84] -> w60
        tunnel: w70 -> [w75 _]
        tunnel: w69 -> [w74 w87]
        tunnel: [w73 w86] -> w64
        tunnel: [w72 w83] -> w61
        tunnel: w58 -> [_ w82]
        tunnel: w55 -> [_ w80]
        frame True {
          # "Interactive (slow)\nCommon IRF"
          n17 = call "AlliGator All ROIs Decay Fit Script.vi"("Lifetime Graph"=w74, "Decay Graph"=w75) -> ("Error Out"=w76:errorcluster, "Message"=w73:string, "All ROIs Decay Fit Script"=w72:T4[])  [unwired: 7 in]
        }
        frame False {
          # "Non-interactive (fast)\nCommon IRF"
          n18 = call "Show Animated Busy Icon with Message and Abort Button.vi"("Already active? (F)"=w81, "Message"=w80, "Target VI reference"=w79) -> ("Error Out"=w78:errorcluster)  [unwired: 16 in]
          n19 = call "AlliGator All ROIs Decay Fit.vi"("error in (no error)"=w78, "Lifetime Graph"=w87, "AlliGator Internal Variables DVR"=w90) -> ("error out"=w88:errorcluster, "Message"=w86:string, "AlliGator Internal Variables DVR"=w89:refnum<data-value>)  [unwired: 6 in]
          n20 = call "Hide Animated Busy Icon with Message and Abort Button.vi"("Already active? (F)"=w81, "Target VI reference"=w79, "Error In"=w88) -> ("Error Out"=w85:errorcluster)  [unwired: 16 in]
          n21 = call "AlliGator Post-Fit Parameter Map Update.vi"("Error In"=w85, "Decay Fit Parameter"=w82) -> ("Error Out"=w84:errorcluster, "Array of Actions"=w83:T4[])  [unwired: 8 in]
        }
      }
      n22 = call-poly "AlliGator Add Action(s) to Stack.vi"("Elements Order in Action Stack (Default: 2 BEFORE 1)"=Alligator_Elements_Order_in_Action_Stack."Enqueue 2 BEFORE 1", "Error In"=w60, "Alligator Queue Element 2"=w61, "Alligator Queue Element 1"=w56) -> ("Error Out"=w59:errorcluster, "Alligator Queue Element 1 (+ 2)"=w62:T4[])  [unwired: 6 in]
    }
    frame "FLI Dataset:All ROIs Phasor Analysis" {
      n23 = Unbundle By Name(w94) -> ("Registered Events Ctrl Refnums.Phasor Graph"=w103:refnum<vi>)
      n24 = call-poly "Variant to Data.vi"("Variant"=w97) -> ("Value"=w104:bool)  [unwired: 8 in]
      n25 = case shown="True" w104 {
        tunnel: w102 -> [w114 w126]
        tunnel: [w113 w126] -> w101
        tunnel: [w108 w138] -> w98
        tunnel: [w105 w137] -> w99
        tunnel: w92 -> [w112 w115]
        tunnel: w91 -> [_ w119]
        tunnel: [w110 w124] -> w95
        tunnel: w103 -> [_ w128]
        tunnel: w96 -> [_ w117]
        tunnel: w100 -> [w106 w121]
        tunnel: w93 -> [_ w118]
        frame True {
          # "Interactive (slow)"
          n26 = call "AlliGator All ROIs Phasor Analysis Script.vi"("Error In"=w112, "AlliGator Internal Variables DVR"=w106) -> ("Error Out"=w109:errorcluster, "All ROIs Analysis Message"=w108:string, "All ROIs Analysis Script"=w107:T4[], "AlliGator Internal Variables DVR"=w105:refnum<data-value>)  [unwired: 6 in]
          n27 = call-poly "AlliGator Add Action(s) to Stack.vi"("Elements Order in Action Stack (Default: 2 BEFORE 1)"=Alligator_Elements_Order_in_Action_Stack."Enqueue 2 BEFORE 1", "Error In"=w109, "Alligator Queue Element 2"=w107, "Alligator Queue Element 1"=w114) -> ("Error Out"=w110:errorcluster, "Alligator Queue Element 1 (+ 2)"=w113:T4[])  [unwired: 6 in]
        }
        frame False {
          w122 = T23 0 items=["Point (.)", "Stepwise Right (--.)", "Line + Point (\\. /)", "Stepwise Left (.--)", "Stepwise Centered (-.-)", "Stepwise Vertical (|.|)", "Line (-)", "Use Previous Plot's Style"] ("Plot Interpolation (Previous Plot's Style)")
          # "Non-interactive (fast)"
          n28 = call "Show Animated Busy Icon with Message and Abort Button.vi"("Already active? (F)"=w119, "Message"=w118, "Target VI reference"=w117, "Error In"=w115) -> ("Error Out"=w116:errorcluster)  [unwired: 15 in]
          n29 = call "XY Graph Try Plot Name.vi"("Error In"=w116, "Plot Name in"="Phasor Plot", "XY Graph Refnum"=w128) -> ("Error Out"=w136:errorcluster, "Plot Name out"=w135:string)  [unwired: 5 in, 2 out]
          n30 = call "AlliGator All ROIs Phasor Analysis.vi"("error in (no error)"=w136, "New Plot Name"=w135, "AlliGator Internal Variables DVR"=w121) -> ("error out"=w127:errorcluster, "Phasor Plot"=w134:cluster{"g Array":dbl[], "s Array":dbl[]}, "AlliGator Internal Variables DVR"=w137:refnum<data-value>, "Message"=w133:string)  [unwired: 3 in, 2 out]
          n31 = call-poly "XY Graph Add Plot(s) with Name(s).vi"("XYGraph Ref in"=w128, "Plot Interpolation (Previous Plot's Style)"=w122, "Plot"=w134, "Plot Name (\"Plot\")"=w135, "error in (no error)"=w127, "Point Style (Dot)"=Plot_Point_Style."Empty Circle") -> ("XY Graph Caption (or Label)"=w129:string, "Plot Name"=w130:string, "error out"=w131:errorcluster)  [unwired: 6 in, 1 out]
          n32 = call "Hide Animated Busy Icon with Message and Abort Button.vi"("Already active? (F)"=w119, "Target VI reference"=w117, "Error In"=w131) -> ("Error Out"=w125:errorcluster)  [unwired: 16 in]
          n33 = Format Into String(format string="\nPlot %s added to %s", initial string=w133, error in=w125, w130, w129) -> (resulting string=w138:string, error out=w124:errorcluster)
        }
      }
    }
    frame "FLI Dataset:All ROIs Average Lifetimes" {
      # "\"FLI Dataset:All ROIs Average Lifetimes\""
      n34 = call "Show Animated Busy Icon with Message and Abort Button.vi"("Already active? (F)"=w139, "Message"=w141, "Target VI reference"=w148) -> ("Error Out"=w150:errorcluster)  [unwired: 16 in]
      n35 = Unbundle By Name(w147) -> ("Registered Events Ctrl Refnums.Lifetime Graph"=w149:refnum<vi>)
      n36 = call "AlliGator All ROIs Average Lifetimes.vi"("error in (no error)"=w150, "Lifetime Graph"=w149, "AlliGator Internal Variables DVR"=w146) -> ("error out"=w140:errorcluster, "Message"=w144:string, "AlliGator Internal Variables DVR"=w143:refnum<data-value>)  [unwired: 6 in]
      n37 = call "Hide Animated Busy Icon with Message and Abort Button.vi"("Already active? (F)"=w139, "Target VI reference"=w148, "Error In"=w140) -> ("Error Out"=w145:errorcluster)  [unwired: 16 in]
    }
    frame "FLI Dataset:All ROIs IRF Extraction" {
      # "All ROIs IRF Extraction"
      n38 = call-poly "Variant to Data.vi"("Variant"=w160) -> ("Value"=w163:bool)  [unwired: 8 in]
      n39 = case shown="False" w163 {
        tunnel: w161 -> [w172 w190]
        tunnel: [w171 w190] -> w157
        tunnel: w158 -> [w170 w189]
        tunnel: [w170 w188] -> w156
        tunnel: w152 -> [w169 w175]
        tunnel: w151 -> [_ w174]
        tunnel: [w167 w187] -> w154
        tunnel: w159 -> [_ w179]
        tunnel: w162 -> [_ w173]
        tunnel: [w164 w178] -> w155
        tunnel: w153 -> [_ w177]
        frame True {
          # "Interactive (slow)"
          n40 = call "AlliGator Script All ROIs IRF Analysis.vi"("Error In"=w169) -> ("Error Out"=w168:errorcluster, "Message"=w164:string, "All ROIs Analysis Script"=w166:T4[])  [unwired: 8 in]
          n41 = call-poly "AlliGator Add Action(s) to Stack.vi"("Elements Order in Action Stack (Default: 2 BEFORE 1)"=Alligator_Elements_Order_in_Action_Stack."Enqueue 2 BEFORE 1", "Error In"=w168, "Alligator Queue Element 2"=w166, "Alligator Queue Element 1"=w172) -> ("Error Out"=w167:errorcluster, "Alligator Queue Element 1 (+ 2)"=w171:T4[])  [unwired: 6 in]
        }
        frame False {
          # "Non-interactive (fast)"
          n42 = call "Show Animated Busy Icon with Message and Abort Button.vi"("Already active? (F)"=w174, "Message"=w177, "Target VI reference"=w173, "Error In"=w175) -> ("Error Out"=w176:errorcluster)  [unwired: 15 in]
          n43 = call "AlliGator All ROIs IRF Analysis.vi"("error in (no error)"=w176, "AlliGator Internal Variables DVR"=w189) -> ("error out"=w186:errorcluster, "# IRFs defined"=w182:i32, "Message"=w178:string, "AlliGator Internal Variables DVR"=w188:refnum<data-value>)  [unwired: 6 in]
          n44 = Unbundle By Name(w179) -> ("Other AlliGator Ctrl Refnums.State Indicators"=w184:refnum<vi>)
          n45 = Not Equal To 0?(x=w182) -> (x != 0?=w181:bool)
          n46 = call "AlliGator Get-Set State Indicators.vi"("# Defined IRFs"=w182, "State Indicators Refnum"=w184, "AlliGator State Indicators List"=AlliGator_State_Indicators_List."Individual IRFs Defined", "Error In"=w186, "ON/OFF"=w181, "Set (T)/Get"=TRUE) -> ("Error Out"=w185:errorcluster)  [unwired: 7 in, 2 out]
          n47 = call "Hide Animated Busy Icon with Message and Abort Button.vi"("Already active? (F)"=w174, "Target VI reference"=w173, "Error In"=w185) -> ("Error Out"=w187:errorcluster)  [unwired: 16 in]
        }
      }
    }
    frame "FLI Dataset:Export Average Lifetime Map as ASCII" {
      # "\"Export Average Lifetime Map as ASCII\""
      n48 = call-poly "Variant to Data.vi"("Variant"=w201) -> ("Value"=w200:bool)  [unwired: 8 in]
      n49 = call "AlliGator Event to String.vi"("AlliGator Q Event"=w193) -> ("String"=w192:string)  [unwired: 8 in]
      n50 = case shown="True" TRUE {
        tunnel: w200 -> [_ w214]
        tunnel: [_ w213] -> w199
        tunnel: w198 -> [_ w205]
        tunnel: w192 -> [_ w212]
        tunnel: w196 -> [_ w211]
        tunnel: w195 -> [w203 w210]
        tunnel: [w203 w208] -> w194
        tunnel: [_ w206] -> w191
        frame False {
          n51 = call "Play Error Sound.vi"() -> ()  [unwired: 27 in, 1 out]
          n52 = One Button Dialog(message="Not yet supported ...") -> ()  [unwired: 1 in, 1 out]
        }
        frame True {
          n53 = call "Show Animated Busy Icon with Message.vi"("Already active? (F)"=w205, "Message"=w212, "Target VI Refnum"=w211) -> ("Error Out"=w209:errorcluster)  [unwired: 8 in]
          n54 = call "AlliGator Export Average Lifetime Map as ASCII.vi"("error in (no error)"=w209, "Dialog?"=w214, "Data Value Reference in"=w210) -> ("error out"=w207:errorcluster, "Message"=w206:string, "Data Value Reference out"=w208:refnum<data-value>)  [unwired: 6 in]
          n55 = call "Hide Animated Busy Icon with Message.vi"("Already active? (F)"=w205, "Error In"=w207, "Target VI reference"=w211) -> ("Error Out"=w213:errorcluster)  [unwired: 8 in]
        }
      }
    }
    frame "FLI Dataset:Export User-Defined Quantity Map as ASCII" {
      # "Export User-Defined Quantity Map as ASCII"
      n56 = call-poly "Variant to Data.vi"("Variant"=w225) -> ("Value"=w224:bool)  [unwired: 8 in]
      n57 = call "AlliGator Event to String.vi"("AlliGator Q Event"=w217) -> ("String"=w216:string)  [unwired: 8 in]
      n58 = case shown="True" TRUE {
        tunnel: w224 -> [_ w238]
        tunnel: [_ w237] -> w223
        tunnel: w222 -> [_ w229]
        tunnel: w216 -> [_ w236]
        tunnel: w220 -> [_ w235]
        tunnel: w219 -> [w227 w234]
        tunnel: [w227 w232] -> w218
        tunnel: [_ w230] -> w215
        frame False {
          n59 = call "Play Error Sound.vi"() -> ()  [unwired: 27 in, 1 out]
          n60 = One Button Dialog(message="Not yet supported ...") -> ()  [unwired: 1 in, 1 out]
        }
        frame True {
          n61 = call "Show Animated Busy Icon with Message.vi"("Already active? (F)"=w229, "Message"=w236, "Target VI Refnum"=w235) -> ("Error Out"=w233:errorcluster)  [unwired: 8 in]
          n62 = call "AlliGator Export User-Defined Quantity Map as ASCII.vi"("error in (no error)"=w233, "Dialog?"=w238, "Data Value Reference in"=w234) -> ("error out"=w231:errorcluster, "Message"=w230:string, "Data Value Reference out"=w232:refnum<data-value>)  [unwired: 6 in]
          n63 = call "Hide Animated Busy Icon with Message.vi"("Already active? (F)"=w229, "Error In"=w231, "Target VI reference"=w235) -> ("Error Out"=w237:errorcluster)  [unwired: 8 in]
        }
      }
    }
    frame "FLI Dataset:Fluorescence Decay Statistics" {
      # "Fluorescence Decay Statistics"
      n64 = call "AlliGator IV Selected Gate Images.vi"("AlliGator IV DVR in"=w243) -> ("Error Out"=w249:errorcluster, "Selected Gate Images"=w250:T24[], "AlliGator IV DVR out"=w251:refnum<data-value>)  [unwired: 8 in]
      n65 = Unbundle By Name(w239) -> ("Other AlliGator Ctrl Refnums.Decay Statistics Bin"=w261:refnum<vi>, "Registered Events Ctrl Refnums.Decay Statistics Graph"=w262:refnum<vi>, "Dataset Control References.Current Data"=w248:refnum<vi>, "Other AlliGator Ctrl Refnums.CPU"=w259:refnum<vi>)
      n66 = property class="DigNum (strict)"(reference=w261) -> ("Value"=w260:i32)  [unwired: 1 in, 2 out]
      n67 = call "Show Animated Busy Icon with Message and Abort Button.vi"("Already active? (F)"=w246, "Message"=w244, "Target VI reference"=w247, "Error In"=w249) -> ("Error Out"=w264:errorcluster)  [unwired: 15 in]
      n68 = call "AlliGator Compute Decay Statistics v2.vi"("Decay Statistics Bin"=w260, "Error In"=w264, "Current Data"=w248, "Image Array"=w250, "Decay Statistics Graph Ref"=w262) -> ("Error Out"=w256:errorcluster, "Message"=w240:string, "Decays Min Values"=w254:sgl[], "Decays Max Values"=w255:sgl[], "Time (s)"=w263:dbl)  [unwired: 2 in]
      n69 = call "Hide Animated Busy Icon with Message and Abort Button.vi"("Already active? (F)"=w246, "Target VI reference"=w247, "Error In"=w256) -> ("Error Out"=w253:errorcluster)  [unwired: 16 in]
      n70 = node(w263) -> (w257:dbl[unit])
      n71 = call "AlliGator IV Decays Max & Min.vi"("Set (T)/Get (F)"=TRUE, "Error In"=w253, "[Decays Min Value]"=w254, "[Decays Max Value]"=w255, "AlliGator IV DVR in"=w251) -> ("Error Out"=w241:errorcluster, "AlliGator IV DVR out"=w242:refnum<data-value>)  [unwired: 3 in, 2 out]
      n72 = property class="DigNum (strict)"(reference=w259, "Value"=w257, "Visible"=TRUE) -> ()  [unwired: 1 in, 2 out]
    }
    frame "FLI Dataset:Channel Arithmetic" {
      # "\"FLI Dataset:Channel Arithmetic\""
      n73 = Variant To Data(type=T17 {"Channel Name"=0, "Channel Arithmetic"=enum."None"} ("Gate Arithmetic Action Parameters"), Variant=w275) -> (data=w271:T17, error out=w269:errorcluster)  [unwired: 1 in]
      n74 = call "Show Animated Busy Icon with Message.vi"("Already active? (F)"=w265, "Message"=w274, "Error In"=w269, "Target VI Refnum"=w277) -> ("Error Out"=w276:errorcluster)  [unwired: 7 in]
      n75 = call "AlliGator Channel Arithmetic Computation.vi"("Error In"=w276, "Channel Arithmetic Action Parameters"=w271, "AlliGator IV DVR in"=w270) -> ("Error Out"=w267:errorcluster, "Message"=w266:string, "AlliGator IV DVR out"=w268:refnum<data-value>)  [unwired: 6 in]
      n76 = call "Hide Animated Busy Icon with Message.vi"("Already active? (F)"=w265, "Error In"=w267, "Target VI reference"=w277) -> ("Error Out"=w273:errorcluster)  [unwired: 8 in]
    }
    frame "FLI Dataset:Get Decay from ROI" {
      # "If no ROI is passed, the current selected ROI is used"
      # "Get Decay from ROI"
      n77 = call "Show Animated Busy Icon with Message.vi"("Already active? (F)"=w282, "Message"=w290, "Target VI Refnum"=w291) -> ("Error Out"=w281:errorcluster)  [unwired: 8 in]
      n78 = Variant To Data(error in=w281, type=T19 {"Global Rectangle"=[], "Contours"=[]} ("ROI Descriptor"), Variant=w288) -> (data=w293:T19, error out=w280:errorcluster)
      n79 = call "Clear Error.vi"("Error In"=w280) -> ("no Error Out"=w279:errorcluster)  [unwired: 8 in]
      n80 = call "AlliGator Get ROI Decay UI.vi"("VI in"=w291, "error in (no error)"=w279, "ROI Descriptor"=w293, "AlliGator Ctrl Refnums"=w287, "AlliGator IV DVR"=w286) -> ("error out"=w292:errorcluster, "Message"=w283:string, "AlliGator IV DVR"=w285:refnum<data-value>)  [unwired: 4 in]
      n81 = call "Hide Animated Busy Icon with Message.vi"("Already active? (F)"=w282, "Error In"=w292, "Target VI reference"=w291) -> ("Error Out"=w284:errorcluster)  [unwired: 8 in]
    }
    frame "FLI Dataset:Logistic Square Gated IRF Characteristics Map" {
      # "Logistic Square Gated IRF Characteristics Map"
      n82 = Unbundle By Name(w295) -> ("Registered Events Ctrl Refnums.Decay Graph"=w304:refnum<vi>)
      n83 = call "AlliGator Get Square Gated IRF Analysis Cursors.vi"("XYGraph in"=w304) -> ("Error Out"=w308:errorcluster, "5 Cursors available?"=w305:bool, "Cursor Names Array"=w306:string[], "Cursor Positions Array"=w307:dbl[])  [unwired: 7 in]
      n84 = case shown="True" w305 {
        tunnel: w302 -> [_ w311]
        tunnel: w296 -> [_ w320]
        tunnel: w308 -> [w310 w314]
        tunnel: w307 -> [_ w319]
        tunnel: w306 -> [_ w318]
        tunnel: [w310 w313] -> w297
        tunnel: w303 -> [_ w317]
        tunnel: w300 -> [w309 w316]
        tunnel: [w309 w315] -> w299
        tunnel: [_ w312] -> w298
        frame False {
        }
        frame True {
          n85 = call "Show Animated Busy Icon with Message and Abort Button.vi"("Already active? (F)"=w311, "Message"=w320, "Target VI reference"=w317, "Error In"=w314) -> ("Error Out"=w322:errorcluster)  [unwired: 15 in]
          n86 = call "AlliGator Logistic Square Gated IRF Characteristics Map.vi"("error in (no error)"=w322, "Cursor Names Array"=w318, "Cursor Positions Array"=w319, "AlliGator Internal Variables DVR"=w316) -> ("error out"=w321:errorcluster, "Message"=w312:string, "AlliGator Internal Variables DVR"=w315:refnum<data-value>)  [unwired: 5 in]
          n87 = call "Hide Animated Busy Icon with Message and Abort Button.vi"("Already active? (F)"=w311, "Target VI reference"=w317, "Error In"=w321) -> ("Error Out"=w313:errorcluster)  [unwired: 16 in]
        }
      }
    }
    frame "FLI Dataset:Multi-ROI Single-Pixel NLSF Analysis" {
      # "Multi-ROI Single-Pixel NLSF Analysis"
      n88 = call "AlliGator NLSF & Phasor Multi-ROI Analysis Dialog.vi"("Dialog Type"=AlliGator_Multi-ROIs_Dialog_Type."Multi-ROIs Single-Pixel NLSF Analysis") -> ("Dataset Loading & Pre-processing Options"=w332:T25, "IRF Loading & Pre-processing Options"=w334:T25, "OK"=w337:bool, "IRF File"=w341:path, "Dataset File"=w340:path, "ROI File"=w339:path, "Decay Fit Parameters to Save"=w338:T43[], "Bins Array"=w335:dbl[], "Results Folder"=w343:path, "error out"=w344:errorcluster)  [unwired: 4 in, 1 out]
      n89 = Unbundle By Name(w328) -> ("Registered Events Ctrl Refnums.Lifetime Graph"=w336:refnum<vi>, "Registered Events Ctrl Refnums.Phasor Graph"=w342:refnum<vi>)
      n90 = case shown="True" w337 {
        tunnel: w327 -> [w347 w367]
        tunnel: [w347 w366] -> w329
        tunnel: w344 -> [w346 w351]
        tunnel: w342 -> [_ w365]
        tunnel: w326 -> [_ w369]
        tunnel: [w346 w368] -> w331
        tunnel: w341 -> [_ w354]
        tunnel: w340 -> [_ w364]
        tunnel: w339 -> [_ w363]
        tunnel: w338 -> [_ w362]
        tunnel: w343 -> [_ w361]
        tunnel: w336 -> [_ w360]
        tunnel: w335 -> [_ w359]
        tunnel: w334 -> [_ w358]
        tunnel: w332 -> [_ w357]
        tunnel: [_ w356] -> w330
        tunnel: w325 -> [w345 w355]
        tunnel: [w345 w350] -> w324
        frame False {
        }
        frame True {
          n91 = Empty String/Path?(string/path=w354) -> (empty?=w353:bool)
          n92 = case shown="True" w353 {
            tunnel: w355 -> [w390 w396]
            tunnel: w351 -> [w389 w395]
            tunnel: [w389 w394] -> w352
            tunnel: [w390 w393] -> w350
            tunnel: [_ w392] -> w348
            tunnel: [TRUE ("Valid Reference?") w391] -> w349
            frame False {
              # "indiv. IRFs"
            }
            frame True {
              # "single IRF"
              n93 = call "AlliGator Check Decay Reference.vi"("Error In"=w395, "AlliGator Internal Variables DVR"=w396) -> ("Error Out"=w394:errorcluster, "Valid Reference?"=w391:bool, "AlliGator Internal Variables DVR"=w393:refnum<data-value>, "Message"=w392:string)  [unwired: 2 in, 4 out]
            }
          }
          n94 = case shown="True" w349 {
            tunnel: w369 -> [_ _]
            tunnel: [w370 w384] -> w368
            tunnel: w367 -> [w371 w387]
            tunnel: [w371 w386] -> w366
            tunnel: w365 -> [_ w385]
            tunnel: w364 -> [_ w383]
            tunnel: w363 -> [_ w382]
            tunnel: w362 -> [_ w381]
            tunnel: w361 -> [_ w380]
            tunnel: w360 -> [_ w379]
            tunnel: w359 -> [_ w378]
            tunnel: w358 -> [_ w377]
            tunnel: w357 -> [_ w376]
            tunnel: [w372 w375] -> w356
            tunnel: w354 -> [_ w374]
            tunnel: w352 -> [w370 w373]
            tunnel: w348 -> [w372 _]
            frame False {
            }
            frame True {
              # "Valid IRF"
              n95 = call "AlliGator Script Multi-ROI Single-Pixel NLSF Analysis.vi"("Alligator Queue Elements in"=w387, "IRF File"=w374, "Dataset File"=w383, "ROI File"=w382, "Decay Fit Parameter to Save"=w381, "Error In"=w373, "Phasor Graph refnum"=w385, "Results Folder"=w380, "Lifetime Graph Refnum"=w379, "Bins Array"=w378, "IRF Loading & Pre-processing Options"=w377, "Dataset Loading & Pre-processing Options"=w376) -> ("Alligator Queue Elements out"=w386:T4[], "Message"=w375:string, "Error Out"=w384:errorcluster)  [unwired: 5 in]
            }
          }
        }
      }
    }
    frame "FLI Dataset:Multi-ROI Single-Pixel Phasor Analysis" {
      # "\"FLI Dataset:Multi-ROI Single-Pixel Phasor Analysis\""
      n96 = Unbundle By Name(w398) -> ("Registered Events Ctrl Refnums.Lifetime Graph"=w409:refnum<vi>, "Registered Events Ctrl Refnums.Phasor Graph"=w414:refnum<vi>)
      n97 = call "Enum to String.vim"("Enum"=w399) -> ("String"=w417:string)
      n98 = call "AlliGator NLSF & Phasor Multi-ROI Analysis Dialog.vi"("Dialog Type"=AlliGator_Multi-ROIs_Dialog_Type."Multi-ROIs Single-Pixel Phasor Analysis", "error in (no error)"=w397) -> ("Dataset Loading & Pre-processing Options"=w406:T25, "IRF Loading & Pre-processing Options"=w408:T25, "OK"=w410:bool, "IRF File"=w413:path, "Dataset File"=w412:path, "ROI File"=w411:path, "Phasor Parameters Scatter Plots"=w405:T44[], "Results Folder"=w415:path, "error out"=w416:errorcluster)  [unwired: 3 in, 2 out]
      n99 = case shown="True" w410 {
        tunnel: w403 -> [w420 w434]
        tunnel: [w420 w433] -> w402
        tunnel: w416 -> [w419 w430]
        tunnel: w414 -> [_ w432]
        tunnel: w417 -> [_ _]
        tunnel: [w419 w431] -> w400
        tunnel: w413 -> [_ w429]
        tunnel: w412 -> [_ w428]
        tunnel: w411 -> [_ w427]
        tunnel: w415 -> [_ w426]
        tunnel: w409 -> [_ w425]
        tunnel: w408 -> [_ w424]
        tunnel: w406 -> [_ w423]
        tunnel: w405 -> [_ w422]
        tunnel: [_ w421] -> w401
        frame False {
        }
        frame True {
          n100 = call "AlliGator Script Multi-ROI Single-Pixel Phasor Analysis.vi"("Alligator Queue Elements in"=w434, "IRF File"=w429, "Dataset File"=w428, "ROI File"=w427, "Error In"=w430, "Phasor Graph refnum"=w432, "Results Folder"=w426, "Lifetime Graph Refnum"=w425, "IRF Loading & Pre-processing Options"=w424, "Phasor Parameters Scatter Plot"=w422, "Dataset Loading & Pre-processing Options"=w423) -> ("Alligator Queue Elements out"=w433:T4[], "Message"=w421:string, "Error Out"=w431:errorcluster)  [unwired: 6 in]
        }
      }
    }
    frame "FLI Dataset:Python Function FLI Dataset Event" {
      # "\"Python Function FLI Dataset Event\""
      n101 = Unbundle By Name(w442) -> ("Dataset Control References.Current Data"=w441:refnum<vi>)
      n102 = call-poly "Variant to Data.vi"("Variant"=w437) -> ("String"=w436:string)  [unwired: 8 in]
      n103 = call "Show Animated Busy Icon with Message.vi"("Already active? (F)"=w435, "Message"=w454, "Target VI Refnum"=w453) -> ("Error Out"=w440:errorcluster)  [unwired: 8 in]
      n104 = property class="Str"(reference=w441, error in=w440) -> (error out=w439:errorcluster, "Value"=w438:string)  [unwired: 1 out]
      n105 = call "AlliGator FLI Dataset Python Function Handler Core.vi"("error in (no error)"=w439, "Current Data"=w438, "Data Value Reference in"=w446, "Item Tag"=w436) -> ("error out"=w444:errorcluster, "Message"=w443:string, "Data Value Reference out"=w445:refnum<data-value>, "Alligator Atomic Action"=w447:T4[])  [unwired: 4 in]
      n106 = call "Hide Animated Busy Icon with Message.vi"("Already active? (F)"=w435, "Error In"=w444, "Target VI reference"=w453) -> ("Error Out"=w450:errorcluster)  [unwired: 8 in]
      n107 = call-poly "AlliGator Add Action(s) to Stack.vi"("Elements Order in Action Stack (Default: 2 BEFORE 1)"=Alligator_Elements_Order_in_Action_Stack."Enqueue 2 BEFORE 1", "Error In"=w450, "Alligator Queue Element 2"=w447, "Alligator Queue Element 1"=w452) -> ("Error Out"=w448:errorcluster, "Alligator Queue Element 1 (+ 2)"=w451:T4[])  [unwired: 6 in]
    }
    frame "FLI Dataset:ROI Analysis" {
      # "\"ROI Analysis\""
      n108 = Unbundle By Name(w468) -> ("Phasor Graph Ctrl Refnums.Phasor Graph Active"=w459:refnum<vi>, "Other AlliGator Ctrl Refnums.Decay Graph Active"=w457:refnum<vi>, "Registered Events Ctrl Refnums.Source Image Display"=w467:refnum<vi>)
      n109 = call "Image Display Get-Set ROI.vi"("Get(F)/Set"=FALSE ("Get(F)/Set(T)"), "Image Display Refnum"=w467) -> ("Error Out"=w464:errorcluster, "Label.Text"=w463:string, "ROI Descriptor out"=w466:T19)  [unwired: 5 in, 2 out]
      n110 = call "Ctrl Refnum to Value (Variant).vi"("Ctl Refnum"=w459) -> ("Value"=w458:variant)  [unwired: 13 in, 1 out]
      n111 = call "Ctrl Refnum to Value (Variant).vi"("Ctl Refnum"=w457) -> ("Value"=w456:variant)  [unwired: 13 in, 1 out]
      n112 = call-poly "Variant to Data.vi"("Variant"=w458) -> ("Value"=w462:bool)  [unwired: 8 in]
      n113 = call-poly "Variant to Data.vi"("Variant"=w456) -> ("Value"=w461:bool)  [unwired: 8 in]
      n114 = Bundle By Name(cluster=T21 {"Image Control Label"="", "ROI Descriptor"={"Global Rectangle"=[], "Contours"=[]}}, "ROI Descriptor"=w466, "Image Control Label"=w463) -> (w472:T21)
      n115 = Compound Arithmetic op=OR(w462, w461) -> (w460:bool)
      n116 = call "AlliGator ROI Analysis Script.vi"("Error In"=w464, "Decay Graph OR Phasor Graph Active?"=w460, "Image ROI"=w472) -> ("Error Out"=w471:errorcluster, "ROI Analysis Script"=w474:T4[])  [unwired: 7 in]
      n117 = call-poly "AlliGator Add Action(s) to Stack.vi"("Elements Order in Action Stack (Default: 2 BEFORE 1)"=Alligator_Elements_Order_in_Action_Stack."Enqueue 2 BEFORE 1", "Error In"=w471, "Alligator Queue Element 2"=w474, "Alligator Queue Element 1"=w477) -> ("Error Out"=w469:errorcluster, "Alligator Queue Element 1 (+ 2)"=w476:T4[])  [unwired: 6 in]
    }
    frame "FLI Dataset:Square Gated IRF Characteristics Map" {
      # "Square Gated IRF Characteristics Map"
      n118 = call "Show Animated Busy Icon with Message and Abort Button.vi"("Already active? (F)"=w478, "Message"=w483, "Target VI reference"=w484) -> ("Error Out"=w487:errorcluster)  [unwired: 16 in]
      n119 = call "AlliGator Square Gated IRF Characteristics Map.vi"("error in (no error)"=w487, "AlliGator Internal Variables DVR"=w482) -> ("error out"=w486:errorcluster, "Message"=w480:string, "AlliGator Internal Variables DVR"=w481:refnum<data-value>)  [unwired: 7 in]
      n120 = call "Hide Animated Busy Icon with Message and Abort Button.vi"("Already active? (F)"=w478, "Target VI reference"=w484, "Error In"=w486) -> ("Error Out"=w479:errorcluster)  [unwired: 16 in]
    }
    frame "FLI Dataset:Tilted Logistic Square Gated IRF Characteristics Map" {
      # "Tilted Logistic Square Gated IRF Characteristics Map"
      n121 = Unbundle By Name(w492) -> ("Registered Events Ctrl Refnums.Decay Graph"=w497:refnum<vi>)
      n122 = call "AlliGator Get Square Gated IRF Analysis Cursors.vi"("XYGraph in"=w497) -> ("Error Out"=w501:errorcluster, "5 Cursors available?"=w498:bool, "Cursor Names Array"=w499:string[], "Cursor Positions Array"=w500:dbl[])  [unwired: 7 in]
      n123 = case shown="True" w498 {
        tunnel: w495 -> [_ w504]
        tunnel: w493 -> [_ w513]
        tunnel: w501 -> [w503 w507]
        tunnel: w500 -> [_ w512]
        tunnel: w499 -> [_ w511]
        tunnel: [w503 w506] -> w490
        tunnel: w496 -> [_ w510]
        tunnel: w491 -> [w502 w509]
        tunnel: [w502 w508] -> w488
        tunnel: [_ w505] -> w489
        frame False {
        }
        frame True {
          n124 = call "Show Animated Busy Icon with Message and Abort Button.vi"("Already active? (F)"=w504, "Message"=w513, "Target VI reference"=w510, "Error In"=w507) -> ("Error Out"=w515:errorcluster)  [unwired: 15 in]
          n125 = call "AlliGator Tilted Square Gated IRF Characteristics Map.vi"("error in (no error)"=w515, "Cursor Names Array"=w511, "Cursor Positions Array"=w512, "AlliGator Internal Variables DVR"=w509) -> ("error out"=w514:errorcluster, "Message"=w505:string, "AlliGator Internal Variables DVR"=w508:refnum<data-value>)  [unwired: 5 in]
          n126 = call "Hide Animated Busy Icon with Message and Abort Button.vi"("Already active? (F)"=w504, "Target VI reference"=w510, "Error In"=w514) -> ("Error Out"=w506:errorcluster)  [unwired: 16 in]
        }
      }
    }
    frame "FLI Dataset:Update Decay Statistics Graph" {
      # "Update Decay Statistics Graph"
      n127 = call "AlliGator IV Decays Max & Min.vi"("Set (T)/Get (F)"=FALSE, "AlliGator IV DVR in"=w521) -> ("Error Out"=w525:errorcluster, "[Decays Min Value]"=w526:sgl[], "[Decays Max Value]"=w527:sgl[], "AlliGator IV DVR out"=w520:refnum<data-value>)  [unwired: 6 in]
      n128 = Unbundle By Name(w522) -> ("Registered Events Ctrl Refnums.Decay Statistics Graph"=w530:refnum<vi>, "Other AlliGator Ctrl Refnums.Decay Statistics Bin"=w529:refnum<vi>)
      n129 = property class="DigNum (strict)"(reference=w529) -> ("Value"=w528:i32)  [unwired: 1 in, 2 out]
      n130 = call "Show Animated Busy Icon with Message.vi"("Already active? (F)"=w516, "Message"=w517, "Error In"=w525, "Target VI Refnum"=w523) -> ("Error Out"=w531:errorcluster)  [unwired: 7 in]
      n131 = call "AlliGator Recompute Decay Statistics Histograms.vi"("Decay Statistics Graph"=w530, "Error In"=w531, "Decay Statistics Bin"=w528, "Decays Min Values"=w526, "Decays Max Values"=w527) -> ("Error Out"=w532:errorcluster)  [unwired: 6 in]
      n132 = call "Hide Animated Busy Icon with Message.vi"("Already active? (F)"=w516, "Error In"=w532, "Target VI reference"=w523) -> ("Error Out"=w518:errorcluster)  [unwired: 8 in]
    }
  }
  "AlliGator IV DVR out" <- w16
  "error out" <- w5
  "Script out" <- w9
  "Alligator Queue Elements" <- w8
  n133 = call "Result Style.vi"() -> ("Default Text Formatting"=w1:T2)
  n134 = call "AlliGator Package Notebook Messages.vi"("Message Formatting"=w1, "Message"=w3, "AlliGator Q Event in"="AlliGator Q Event in") -> ("[Notebook Message]"=→"[Notebook Message]":T1[])  [unwired: 8 in]
